vi "CRYMessages Editor.vi"() -> ()   [LabVIEW 2013]
uses:
  Typedef Control/CRYMessages Cluster.ctl
  <vilib>/Utility/miscctls.llb/LVBoundsTypeDef.ctl
  Typedef Control/CRYText Format.ctl
  CRYProject/CRYProject Editor Global.vi
  CRYWindow/SubVI/CRYMain Sub Window Global.vi
  CRYMainGlobal.vi
  CRYStepSetup/CRYStepSetup Global.vi
panel:
  in  "Digital IO Update":bool caption="对话"
  out "Message Cluster Bk":T1={"Name"="Default", "Type"=0, "Command Msg"="<Enter message or command here>", "Flags"=0, "Dialog?"=FALSE, "Numeric?"=FALSE, "Wait?"=FALSE, "Pause [ms]"=0, "pattern"=0, "Address"="", "Operation"=0, "bytes"=0, "Line selected"=0, "RS232 Func"=0, "Serial Ctrl lines"=0, "Interf #"=0, "GPIB func"=0, "GPIB cmd"=0, "GPIB rem en"=FALSE, "GPIB term"=0, "Curves generated"=[], "Units"={"unit"="", "dB ref"=0.0, "axis"=0, "data"=0, "Common dB ref."=1}, "Axis"=0, "Default Value"=0.0, "Message Tilte"="", "Port #"=0, "Print Unit"="", "Text Format"={"Size"=0, "Plain"=FALSE, "Bold"=FALSE, "Italic"=FALSE, "Underline"=FALSE, "Strikethrough"=FALSE, "Color"=0, "Font"=""}, "Help"="", "Tab Value"=enum."Setting", "pattern 2"=0, "Line selected 2"=0, "H_Bits"=[], "G_Bits"=[]} {"pattern 2" format="%.0b"; "Units"."Common dB ref." items=["dB", "dBSPL", "dBPa", "dBV", "dBm", "dBu", "dBFS"]; "Units"."dB ref" format="%.2f"; "pattern" format="%.0b"; "Flags" items=["Pass", "Fail"]}
  out "EndFlag":bool
  in  "Add Lib":bool caption="Apply"
  in  "AddStep":bool
  in  "Board Tab":enum32{"Page 1"}(tab)
  in  "Cancel":bool caption="Apply"
  in  "OK":bool caption="Apply"
  in  "Main Tab":enum32{"Setting", "Help"}(tab)
  in  "Setting":bool caption="Apply"
  in  "Line selected 2":T2={"Line"=TRUE, "Line"=TRUE, "Line"=TRUE, "Line"=TRUE, "Line"=TRUE, "Line"=TRUE, "Line"=TRUE, "Line"=TRUE} caption="Port H"
  out "Pattern 2":T3
  in  "Wait unit":string
  in  "RS-232 Func":u16(ring) caption="功能" items=["Write/Read Message", "Set Control Lines", "Read Control Lines"]
  in  "Format Text":bool
  in  "Serial Ctrl line":u16(slide) caption="Type 2"
  in  "Serial Ctrl line Read":u16(slide) caption="Type 2"
  in  "Remote Enable":bool caption="远程启用"
  in  "Command":u16(ring) caption="命令" items=["Device Clear", "Selected Device Clear", "Group Execute Trigger", "Go To Local", "Local Lockout", "Unlisten"]
  out "Interface Type":u16(ring) items=["IEEE-488", "RS-232", "Footswitch", "Buzzer"]
  in  "GPIB Function":u16(ring) caption="功能" items=["Write/Read Message", "Interface Message", "Serial Poll", "Wait for Service Request"]
  in  "Msg. term.":i32(ring) caption="项目" items=["EOI", "CR, EOI", "LF, EOI", "CR, LF, EOI", "CR", "LF", "CR, LF", "none"]
  in  "Address":i32=1 caption="地址" min=1 max=31 step=1
  in  "Bytes":i32 caption="位数"
  in  "Line selected":T2={"Line"=TRUE, "Line"=TRUE, "Line"=TRUE, "Line"=TRUE, "Line"=TRUE, "Line"=TRUE, "Line"=TRUE, "Line"=TRUE} caption="Port G"
  out "Pattern":T3
  in  "Dlg Def Val":u16(slide) caption="默认值"
  in  "Operation":i32(slide)
  in  "Dialog":bool caption="对话"
  in  "Numeric":bool caption="数字"
  in  "Wait":bool caption="等待"
  in  "Flags":u16(slide)=1
  in  "Command Msg":string="NO ELECTRICAL SIGNAL DETECTED!\nCheck wiring and connections."
  in  "Type":u16(slide)
  in  "Message Title":string caption="消息标题"
  out "DIO direction":bool=TRUE
  in  "Port":i32(ring) caption="端口"
  in  "No.":u8(ring) caption="Port"
  in  "Timeout":i32 caption="暂停" min=0 max=999999 step=1
  in  "Units Tab":enum32{"Page 1"}(tab)
  in  "Axis":u16(slide) caption="轴" scale=0.0..2.0
  out "Units":string caption="单位"
  in  "Default Value":dbl caption="默认值" format="%#.6p"
  in  "Unit Control":bool caption="Unit..."
  out "Settings":bool caption="设置"
  out "Message":bool caption="消息"
  in  "Help":string
  in  "Apply":bool
  in  "Save As...":bool caption="Apply"
  in  "Revert":bool caption="Apply"
  in  "Load...":bool caption="Apply"
  out "Interface Name":u16[](array[numeric])
  in  "Text Format":T4
  in  "Units Cluster":T5={"unit"="", "dB ref"=0.0, "axis"=0, "data"=0, "Common dB ref."=1} {"Common dB ref." items=["dB", "dBSPL", "dBPa", "dBV", "dBm", "dBu", "dBFS"]; "dB ref" format="%.2f"}
  out "DIO Array":bool[](array[boolean])
  in  "Channel":i32=-1
  in  "Calibration in":string
  in  "Hardware in":string
  in  "Load Test":bool
  out "Proper VI No":i32
  out "VIMiniumBound":T6
  out "Message Cluster":T1={"Name"="Default", "Type"=0, "Command Msg"="<Enter message or command here>", "Flags"=0, "Dialog?"=FALSE, "Numeric?"=FALSE, "Wait?"=FALSE, "Pause [ms]"=0, "pattern"=0, "Address"="", "Operation"=0, "bytes"=0, "Line selected"=0, "RS232 Func"=0, "Serial Ctrl lines"=0, "Interf #"=0, "GPIB func"=0, "GPIB cmd"=0, "GPIB rem en"=FALSE, "GPIB term"=0, "Curves generated"=[], "Units"={"unit"="", "dB ref"=0.0, "axis"=0, "data"=0, "Common dB ref."=1}, "Axis"=0, "Default Value"=0.0, "Message Tilte"="", "Port #"=0, "Print Unit"="", "Text Format"={"Size"=0, "Plain"=FALSE, "Bold"=FALSE, "Italic"=FALSE, "Underline"=FALSE, "Strikethrough"=FALSE, "Color"=0, "Font"=""}, "Help"="", "Tab Value"=enum."Setting", "pattern 2"=0, "Line selected 2"=0, "H_Bits"=[], "G_Bits"=[]} {"pattern 2" format="%.0b"; "Units"."Common dB ref." items=["dB", "dBSPL", "dBPa", "dBV", "dBm", "dBu", "dBFS"]; "Units"."dB ref" format="%.2f"; "pattern" format="%.0b"; "Flags" items=["Pass", "Fail"]}
  in  "stop":bool
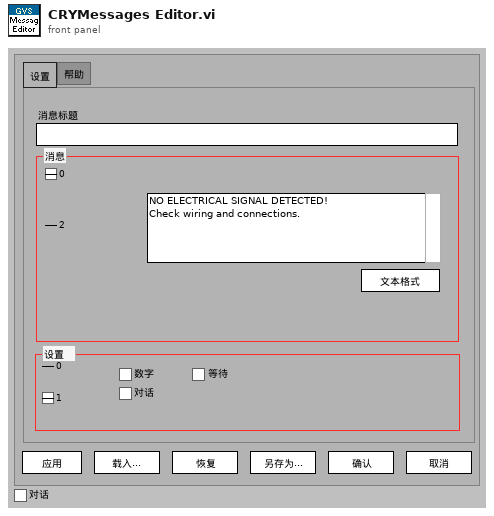
[diagram p1: front panel]
types:
  T1 = typedef "CRYMessages Cluster.ctl" = cluster{"Name":string, "Type":u16, "Command Msg":string, "Flags":u16, "Dialog?":bool, "Numeric?":bool, "Wait?":bool, "Pause [ms]":i32, "pattern":u32, "Address":string, "Operation":i32, "bytes":i32, "Line selected":u32, "RS232 Func":u16, "Serial Ctrl lines":u16, "Interf #":u8, "GPIB func":u16, "GPIB cmd":u16, "GPIB rem en":bool, "GPIB term":i32, "Curves generated":string[], "Units":cluster{"unit":string, "dB ref":dbl, "axis":u16, "data":u16, "Common dB ref.":u16}, "Axis":u16, "Default Value":dbl, "Message Tilte":string, "Port #":i32, "Print Unit":string, "Text Format":cluster{"Size":u32, "Plain":bool, "Bold":bool, "Italic":bool, "Underline":bool, "Strikethrough":bool, "Color":u32, "Font":string}, "Help":string, "Tab Value":enum32{"Setting", "Help"}, "pattern 2":u32, "Line selected 2":u32, "H_Bits":cluster{"Bits":string[], "Invert":bool, "All":bool}[], "G_Bits":cluster{"Bits":string[], "Invert":bool, "All":bool}[]}
  T2 = cluster{"Line":bool, "Line":bool, "Line":bool, "Line":bool, "Line":bool, "Line":bool, "Line":bool, "Line":bool}
  T3 = cluster{"0":bool, "1":bool, "2":bool, "3":bool, "4":bool, "5":bool, "6":bool, "7":bool}
  T4 = typedef "CRYText Format.ctl" = cluster{"Size":u32, "Plain":bool, "Bold":bool, "Italic":bool, "Underline":bool, "Strikethrough":bool, "Color":u32, "Font":string}
  T5 = cluster{"unit":string, "dB ref":dbl, "axis":u16, "data":u16, "Common dB ref.":u16}
  T6 = typedef "LVBoundsTypeDef.ctl" = cluster{"Width":u32, "Height":u32}
  T7 = typedef "CRYStep.ctl" = cluster{"No.VI":i32, "Category":string, "StepName":string, "Seq setup flattened":string, "Comment":string, "Steps config.":bool[], "Jump config":i32[], "Start":dbl, "Increment":dbl, "Name":string, "Unit":string, "Y data":u16, "Y prefix":string, "Y dB ref":dbl, "Y unit":string, "Repeat State Array":cluster{"Start":dbl, "Increment":dbl, "Count":i32, "Num":i32}[]}
  T8 = typedef "CRYHardware.ctl" = cluster{"Name":string, "Analog I/O":u16, "Digital I/O":u16, "Channels":u8, "Dig Dev ID":u8, "N ports":u8, "Interface":u32, "Dig I/O Ports":cluster{"port #":i16, "width":i16, "direction":i32}[], "Interf settings":cluster{"Type":u16, "COM Port":u8, "Baud rate":u32, "Data bits":u32, "Parity":u16, "Stop bits":u16, "Flow control":u16, "Dev ID IEEE":u8}[], "N interfs":i32, "udev SNs":i16[], "udev enable":bool, "Channel Array":T9[], "Cal sequence":string, "SelectedIn":u16, "SelectedOut":u16, "SelectedTab":u16, "State":bool, "Help":string, "Advanced":bool, "In Audio Driver":u16, "Out Audio Driver":u16}
  T9 = typedef "CRYHardware Channel Info.ctl" = cluster{"ID":i32, "Name":string, "Digital":bool, "Input":bool, "Device Name":string, "Hardware Ch ID":u8, "Vmax (V)":dbl, "Latency (samples)":dbl, "Sampling Rate (Hz)":u32, "Bit Depth":u32, "Anti-aliasing Factor (%fs)":sgl, "DAQmx Channel":tag, "term config":i32, "Coupling":i32, "IEPE en":bool, "ASIOChannel Name":string, "Audio Driver":u16, "ASIOChannel Index":u8}
  T10 = cluster{"port #":i16, "width":i16, "direction":i32}[]
  T11 = cluster{"Type":u16, "COM Port":u8, "Baud rate":u32, "Data bits":u32, "Parity":u16, "Stop bits":u16, "Flow control":u16, "Dev ID IEEE":u8}[]
  T12 = enum16{"OK", "Yes", "YesNo", "YesNoCancel", "ReplaceAppend"}
  T13 = enum8{"Enabled", "Disabled", "Disabled and Grayed Out"}
  T14 = cluster{"Bits":string[], "Invert":bool, "All":bool}[]
  T15 = cluster{"Load Test":bool, "Format Text":bool, "Unit Control":bool, "Apply":bool, "Add Lib":bool, "OK":bool, "Cancel":bool, "Setting":bool}
  T16 = cluster{"Size":u32, "Plain":bool, "Bold":bool, "Italic":bool, "Underline":bool, "Strikethrough":bool, "Color":u32, "Font":string}
  T17 = cluster{"Boolean array[0]":bool, "Boolean array[1]":bool, "Boolean array[2]":bool, "Boolean array[3]":bool, "Boolean array[4]":bool, "Boolean array[5]":bool, "Boolean array[6]":bool, "Boolean array[7]":bool}
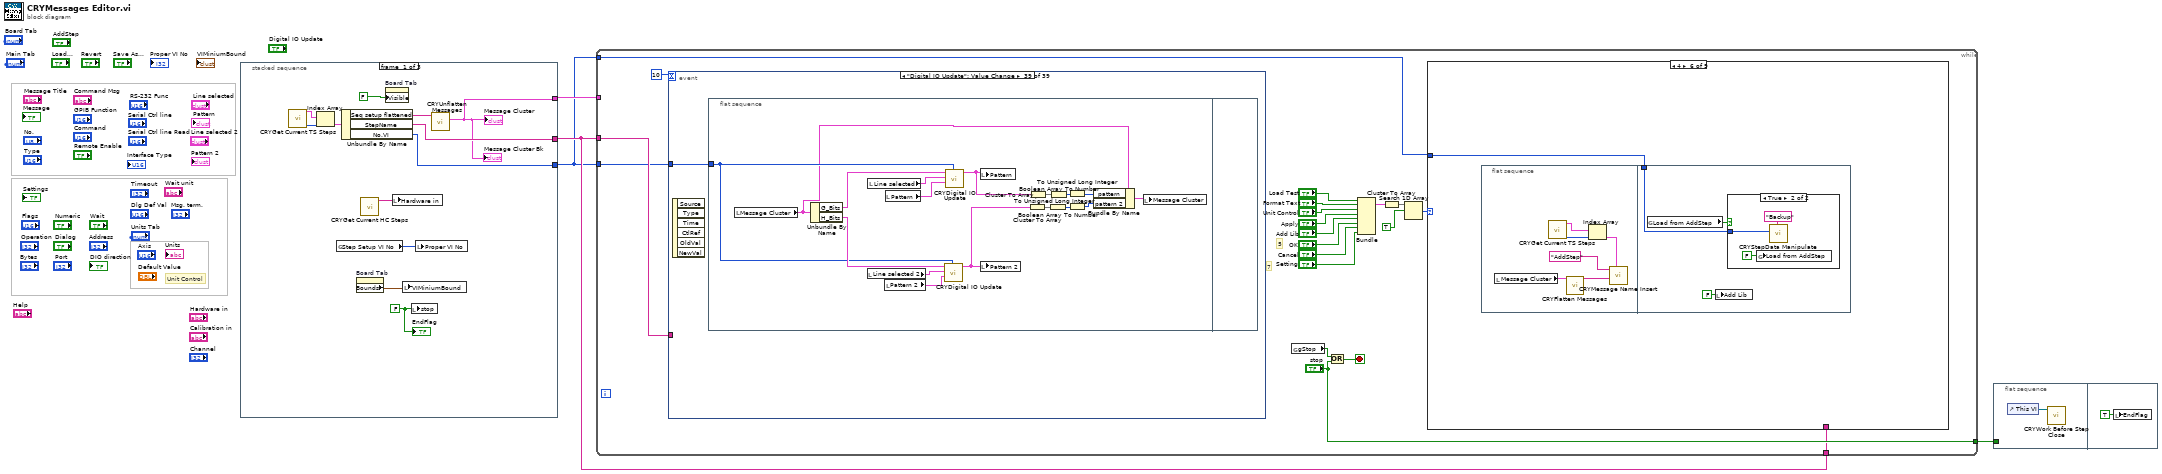
[diagram p0: block diagram]
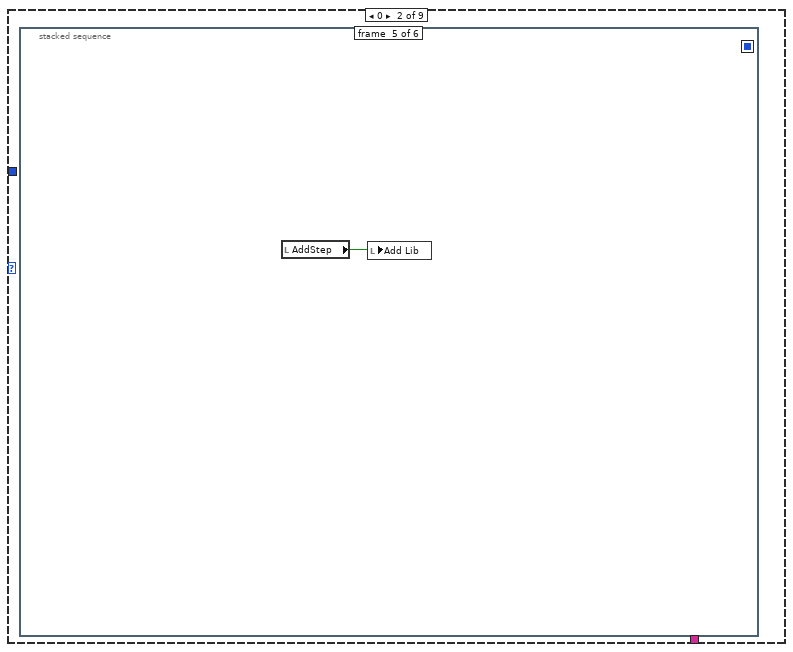
[diagram p3: hidden frame]
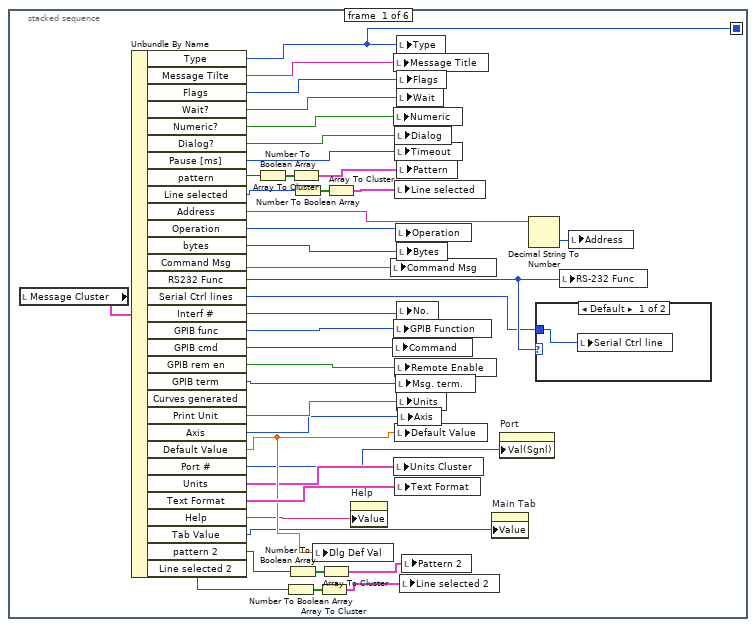
[diagram p4: hidden frame]
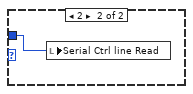
[diagram p5: hidden frame]
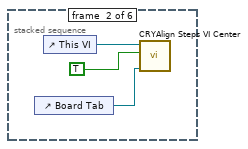
[diagram p6: hidden frame]
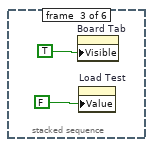
[diagram p7: hidden frame]
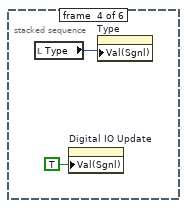
[diagram p8: hidden frame]
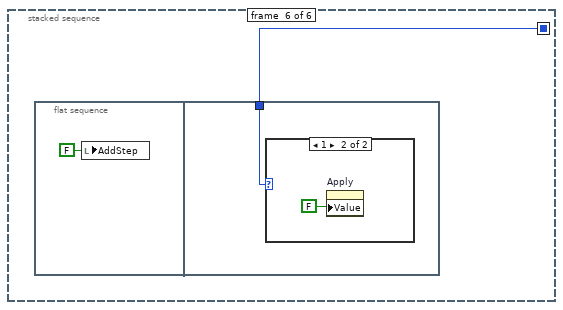
[diagram p9: hidden frame]
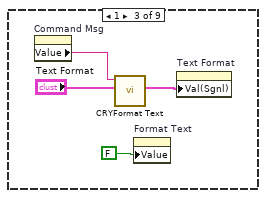
[diagram p11: hidden frame]
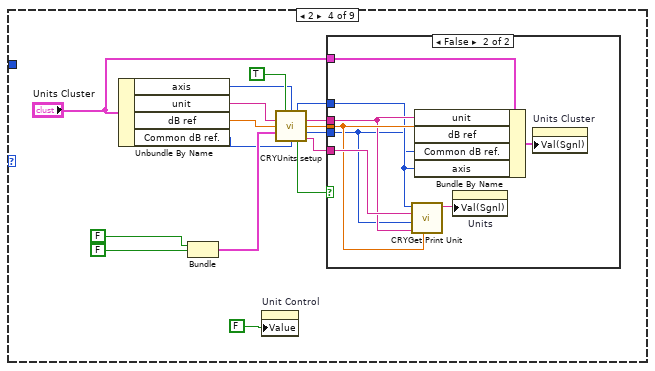
[diagram p12: hidden frame]
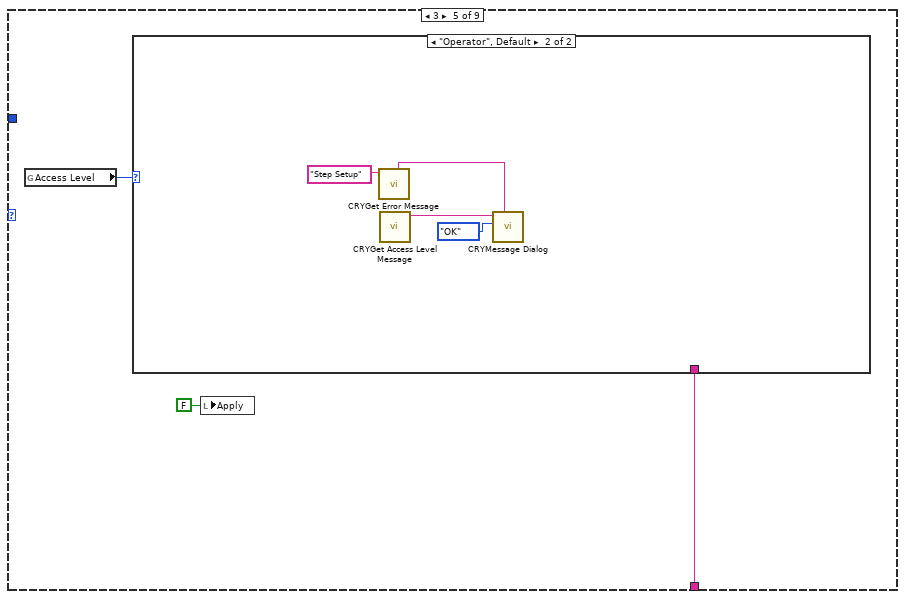
[diagram p14: hidden frame]
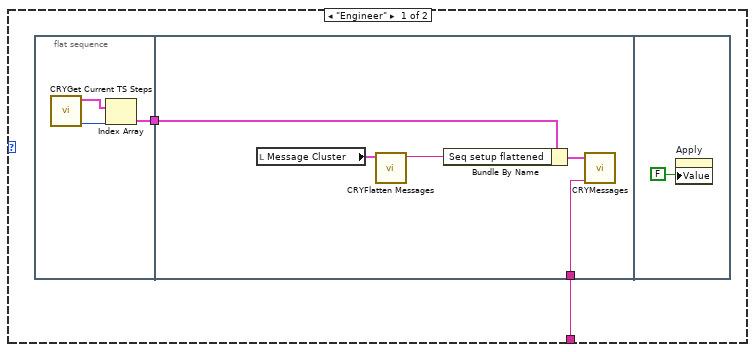
[diagram p15: hidden frame]
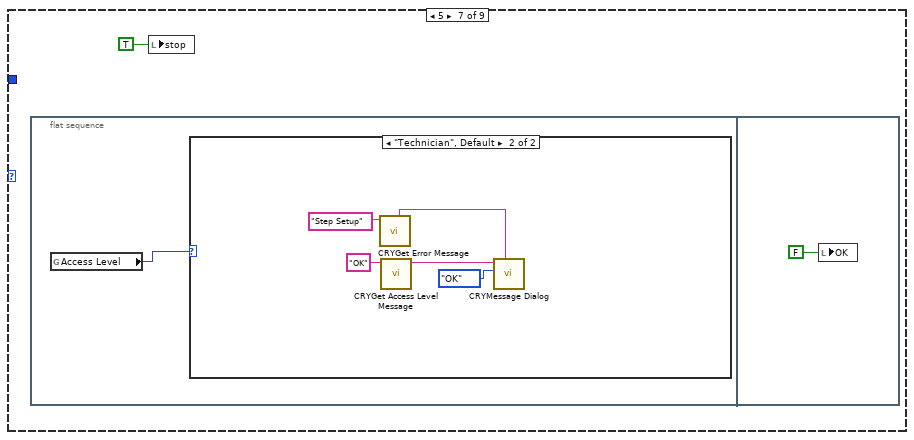
[diagram p17: hidden frame]
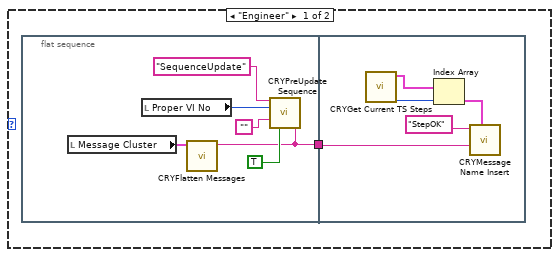
[diagram p18: hidden frame]
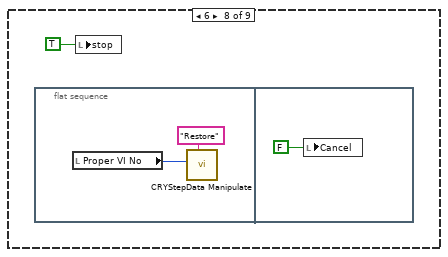
[diagram p19: hidden frame]
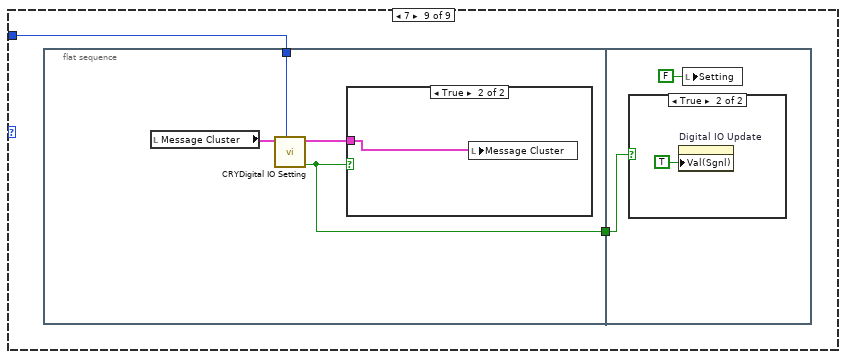
[diagram p20: hidden frame]
diagram:
  # "Unit Control"
  n1 = stacked-sequence {
    tunnel: [w7 _ _] -> w4
    tunnel: [w8 _ _] -> w2
    tunnel: [w5 _ _] -> w1
    frame #0 {
      w6 = FALSE ("stop")
      n2 = call "CRYGet Current TS Steps.vi"() -> ("SelectStepNumber in Tree"=w12:i32, "Steps"=w13:T7[])  [unwired: 1 in, 9 out]
      n3 = Index Array(array=w13, index=w12) -> (element=w16:T7)
      n4 = global read "CRYProject Editor Global.vi" "Step Setup VI No"() -> (w14:i32)
      n5 = Unbundle By Name(w16) -> ("Seq setup flattened"=w15:string, "StepName"=w8:string, "No.VI"=w5:i32)
      n6 = property on="Board Tab" class="TabCtl (strict)"() -> ("Bounds"=w10:T6)  [unwired: 2 in, 2 out]
      n7 = call "CRYGet Current HC Steps.vi"() -> ("Hardware setup flattened Out"=w9:string)  [unwired: 10 in, 1 out]
      n8 = property on="Board Tab" class="TabCtl (strict)"("Visible"=FALSE) -> ()  [unwired: 2 in, 2 out]
      n9 = local write "Hardware in"(w9) -> ()
      n10 = local write "VIMiniumBound"(w10) -> ()
      n11 = local write "stop"(w6) -> ()
      n12 = local write "Proper VI No"(w14) -> ()
      n13 = call "CRYUnflatten Messages.vi"("Unflatten Messages"=w15) -> ("Messages"=w7:T1)  [unwired: 10 out]
      "Message Cluster" <- w7
      "Message Cluster Bk" <- w7
      "EndFlag" <- w6
    }
    frame #1 {
      w19 = FALSE ("Visible")
      n14 = local read "Hardware in"() -> (w26:string)
      n15 = call "CRYUnflatten SoundCard.vi"("Flatten SoundCard"=w26) -> ("SoundCard"=w29:T8)  [unwired: 10 out]
      n16 = local write "Wait unit"("ms" ("Wait unit")) -> ()
      n17 = Unbundle By Name(w29) -> ("N ports"=w28:u8, "Dig I/O Ports"=w23:T10, "N interfs"=w20:i32, "Interf settings"=w25:T11)
      n18 = property on="Unit Control" class="Bool (strict)"("Value"=w19) -> ()  [unwired: 2 in, 2 out]
      n19 = local write "Default Value"(0.0 ("Default Value")) -> ()
      n20 = for {
        N: w20 -> [_]
        tunnel: [w32] -> w27 mode=indexing
        tunnel: w25 -> [w31] mode=indexing
        tunnel: [w30] -> w24 mode=indexing
        i -> [w34]
        n21 = Increment(x=w34) -> (x+1=w33:i32)
        n22 = Unbundle By Name(w31) -> ("Type"=w30:u16)
        n23 = Number To Decimal String(number=w33) -> (decimal integer string=w32:string)  [unwired: 1 out]
      }
      "Interface Name" <- w24
      n24 = for {
        N: w28 -> [_]
        tunnel: [w38] -> w21 mode=indexing
        tunnel: w23 -> [w36] mode=indexing
        tunnel: [w35] -> w22 mode=indexing
        i -> [w40]
        n25 = Increment(x=w40) -> (x+1=w39:i32)
        n26 = Unbundle By Name(w36) -> ("direction"=w37:i32)
        n27 = Number To Decimal String(number=w39) -> (decimal integer string=w38:string)  [unwired: 1 out]
        n28 = Not Equal To 0?(x=w37) -> (x != 0?=w35:bool)
      }
      "DIO Array" <- w22
      n29 = property on="Format Text" class="Bool (strict)"("Value"=w19) -> ()  [unwired: 2 in, 2 out]
      n30 = property on="Apply" class="Bool (strict)"("Value"=w19) -> ()  [unwired: 2 in, 2 out]
      n31 = property on="No." class="Ring (strict)"("Strings []"=w27) -> ()  [unwired: 2 in, 2 out]
      n32 = property on="Port" class="Ring (strict)"("Strings []"=w21) -> ()  [unwired: 2 in, 2 out]
    }
    frame #2 {
      n33 = property on="Load Test" class="Bool (strict)"("Value"=TRUE ("Load Test")) -> ()  [unwired: 2 in, 2 out]
    }
  }
  n34 = while {
    tunnel: w4 -> [_]
    tunnel: ["stop"] -> w3
    tunnel: w2 -> [w49]
    tunnel: w2 -> [w48]
    tunnel: w1 -> [w43]
    tunnel: w1 -> [w42]
    stop <- w52 stop-if-true
    # "7"
    # "5"
    n35 = event shown="[38] \"Digital IO Update\": Value Change" {
      selector: _ -> [_ _ _ _ _ _ _ _ _ _ _ _ _ _ _ _ _ _ _ _ _ _ _ _ _ _ _ _ _ _ _ _ _ _ _ _ _ _ _]
      dyn-events: _ -> [_ _ _ _ _ _ _ _ _ _ _ _ _ _ _ _ _ _ _ _ _ _ _ _ _ _ _ _ _ _ _ _ _ _ _ _ _ _ _]
      timeout: 10 -> [_ _ _ _ _ _ _ _ _ _ _ _ _ _ _ _ _ _ _ _ _ _ _ _ _ _ _ _ _ _ _ _ _ _ _ _ _ _ _]
      tunnel: w49 -> [_ _ _ _ _ _ w263 w309 w321 _ w346 _ w382 w402 _ _ _ _ _ _ _ _ _ _ _ _ _ _ w497 _ _ _ _ _ _ _ _ _ _]
      tunnel: w43 -> [_ _ _ _ _ _ _ _ _ _ _ _ _ _ _ _ _ _ _ _ _ _ _ _ _ _ _ _ _ _ _ _ _ _ _ _ _ _ w560]
      event Timeout {
        n36 = event-data() -> ()  [unwired: 3 out]
      }
      event Pane Size {
        n37 = event-data() -> ()  [unwired: 7 out]
        n38 = control-ref of="Board Tab"() -> (w209:refnum<vi>)
        n39 = control-ref of="This VI"() -> (w211:refnum<vi>)
        n40 = call "CRYAlign Steps VI Center.vi"("Tab2"=w209, "Input/Output"=TRUE, "VIRef"=w211) -> ()  [unwired: 1 in, 8 out]
      }
      event "Load...": Value Change {
        n41 = event-data() -> ("CtlRef"=w212:refnum<vi>)  [unwired: 6 out]
        n42 = property on="Load Test" class="Bool (strict)"() -> ("Value"=w214:bool)  [unwired: 2 in, 2 out]
        n43 = property class="Bool (strict)"(reference=w212, "Value"=FALSE) -> ()  [unwired: 1 in, 2 out]
        n44 = case shown="False" w214 {
          frame False {
            n45 = global read "CRYMainGlobal.vi" "Steps path"() -> (w219:path)
            n46 = local read "Proper VI No"() -> (w215:i32)
            n47 = Build Path(base path=w219, name or relative path="CRYMessages") -> (appended path=w220:path)
            n48 = call "CRYStep Read.vi"("Category Name"="Messages" ("Step File Name"), "Proper VI No"=w215, "Step File Path"=w220) -> ("status"=w221:bool, "selected path"=w216:path, "Flatten Step"=w222:string)  [unwired: 1 in, 3 out]
            n49 = case shown="True" w221 {
              tunnel: w222 -> [_ w224]
              tunnel: w216 -> [_ w225]
              tunnel: w215 -> [_ w223]
              frame False {
              }
              frame True {
                n50 = call "CRYUnflatten Messages.vi"("Unflatten Messages"=w224) -> ("Error?"=w226:bool, "Messages"=w227:T1)  [unwired: 9 out]
                n51 = case shown="False" w226 {
                  tunnel: w227 -> [w231 _]
                  tunnel: w225 -> [w230 _]
                  tunnel: w224 -> [w229 _]
                  tunnel: w223 -> [w228 _]
                  frame False {
                    n52 = flat-sequence {
                      tunnel: w231 -> [w243]
                      tunnel: w230 -> [w239]
                      tunnel: w229 -> [w237]
                      tunnel: w228 -> [w238]
                      frame #0 {
                        n53 = local write "Message Cluster"(w243) -> ()
                        n54 = Strip Path(path=w239) -> (name=w233:string)  [unwired: 1 out]
                        n55 = Reverse String(1:w233) -> (0:w235:string)
                        n56 = Match Pattern(string=w235, regular expression="[.]") -> (after substring=w236:string)  [unwired: 4 out]
                        n57 = Reverse String(1:w236) -> (0:w232:string)
                        n58 = call "CRYPreUpdate Sequence.vi"("EventName"="Load", "StepName Arg3"=w232, "Proper VI No"=w238, "Project View Step Name Identifier Arg1"="", "Step flattened Arg2"=w237, "AllChangeFlg"=TRUE ("Name/Identifier")) -> ()  [unwired: 10 in]
                      }
                      frame #1 {
                        n59 = local write "Load Test"(TRUE ("Load Test")) -> ()
                      }
                    }
                  }
                  frame True {
                  }
                }
              }
            }
          }
          frame True {
          }
        }
      }
      event "Save As...": Value Change {
        w247 = "Messages" ("Step File Name")
        n60 = event-data() -> ("CtlRef"=w245:refnum<vi>)  [unwired: 6 out]
        n61 = property class="Bool (strict)"(reference=w245, "Value"=FALSE) -> ()  [unwired: 1 in, 2 out]
        n62 = local read "Message Cluster"() -> (w255:T1)
        n63 = global read "CRYMainGlobal.vi" "Steps path"() -> (w248:path)
        n64 = call "CRYFlatten Messages.vi"("Messages"=w255) -> ("Flatten Messages String"=w249:string)  [unwired: 10 out]
        n65 = local read "Proper VI No"() -> (w250:i32)
        n66 = Build Path(base path=w248, name or relative path="CRYMessages") -> (appended path=w252:path)
        n67 = call "CRYStep Write.vi"("StepIdentifier"="", "Default"=FALSE, "Proper VI No"=w250, "Category Name"=w247, "Step File Path"=w252, "Step flattened"=w249, "Step File Name"=w247) -> ()  [unwired: 1 in, 4 out]
      }
      event "Revert": Value Change {
        n68 = event-data() -> ("CtlRef"=w257:refnum<vi>)  [unwired: 6 out]
        n69 = flat-sequence {
          frame #0 {
            n70 = local read "Message Cluster Bk"() -> (w258:T1)
            n71 = local write "Message Cluster"(w258) -> ()
          }
          frame #1 {
            n72 = local write "Load Test"(TRUE ("Load Test")) -> ()
          }
        }
        n73 = property class="Bool (strict)"(reference=w257, "Value"=FALSE) -> ()  [unwired: 1 in, 2 out]
      }
      event Panel Close {
        n74 = event-data() -> ()  [unwired: 5 out]
        n75 = control-ref of="This VI"() -> (w261:refnum<vi>)
        n76 = local write "Cancel"(TRUE ("Cancel")) -> ()
        n77 = call "CRYWork Before Step Close.vi"("StepVI Ref"=w261) -> ()  [unwired: 11 in]
      }
      event "Type": Value Change {
        n78 = event-data() -> ("NewVal"=w264:u16)  [unwired: 6 out]
        n79 = local read "Interface Type"() -> (w271:u16)
        n80 = local read "RS-232 Func"() -> (w270:u16)
        n81 = local read "Operation"() -> (w269:i32)
        n82 = local read "Numeric"() -> (w267:bool)
        n83 = local read "Dialog"() -> (w268:bool)
        n84 = local read "GPIB Function"() -> (w272:u16)
        n85 = case shown="1" w264 {
          tunnel: [FALSE TRUE FALSE] -> w262
          frame 0, Default {
            w275 = FALSE
            w291 = TRUE ("Visible")
            n86 = local read "Numeric"() -> (w289:bool)
            n87 = local read "Dialog"() -> (w290:bool)
            n88 = property on="DIO direction" class="Bool (strict)"("Visible"=w275) -> ()  [unwired: 2 in, 2 out]
            n89 = property on="Pattern" class="Clust (strict)"("Visible"=w275) -> ()  [unwired: 2 in, 2 out]
            n90 = property on="Command Msg" class="Str"("Visible"=w291) -> ()  [unwired: 2 in, 2 out]
            n91 = property on="Flags" class="Slide (strict)"("Visible"=w291) -> ()  [unwired: 2 in, 2 out]
            n92 = Equal?(x=w290, y=FALSE) -> (x = y?=w284:bool)
            n93 = Equal?(x=w289, y=FALSE) -> (x = y?=w285:bool)
            n94 = property on="Line selected" class="Clust (strict)"("Visible"=w275) -> ()  [unwired: 2 in, 2 out]
            n95 = property on="Wait" class="Bool (strict)"("Visible"=w291) -> ()  [unwired: 2 in, 2 out]
            n96 = Not(x=w285) -> (.not. x?=w283:bool)
            n97 = property on="Port" class="Ring (strict)"("Visible"=w275) -> ()  [unwired: 2 in, 2 out]
            n98 = Not(x=w284) -> (.not. x?=w286:bool)
            n99 = property on="Format Text" class="Bool (strict)"("Visible"=w291) -> ()  [unwired: 2 in, 2 out]
            n100 = And(x=w284, y=w285) -> (x .and. y?=w279:bool)
            n101 = And(x=w286, y=w285) -> (x .and. y?=w278:bool)
            n102 = And(x=w284, y=w283) -> (x .and. y?=w277:bool)
            n103 = property on="Command" class="Ring (strict)"("Visible"=w275) -> ()  [unwired: 2 in, 2 out]
            n104 = property on="No." class="Ring (strict)"("Visible"=w275) -> ()  [unwired: 2 in, 2 out]
            n105 = property on="Numeric" class="Bool (strict)"("Visible"=w291) -> ()  [unwired: 2 in, 2 out]
            n106 = Bundle(w279, w278, w277) -> (w281:cluster{bool, bool, bool})  [unwired: 1 out]
            n107 = property on="Remote Enable" class="Bool (strict)"("Visible"=w275) -> ()  [unwired: 2 in, 2 out]
            n108 = property on="Interface Type" class="Ring (strict)"("Visible"=w275) -> ()  [unwired: 2 in, 2 out]
            n109 = Cluster To Array(cluster=w281) -> (array=w280:bool[])
            n110 = property on="Dialog" class="Bool (strict)"("Visible"=w291) -> ()  [unwired: 2 in, 2 out]
            n111 = Search 1D Array(1D array=w280, element=TRUE) -> (index of element=w276:i32)  [unwired: 1 out]
            n112 = property on="RS-232 Func" class="Ring (strict)"("Visible"=w275) -> ()  [unwired: 2 in, 2 out]
            n113 = property on="GPIB Function" class="Ring (strict)"("Visible"=w275) -> ()  [unwired: 2 in, 2 out]
            n114 = case shown="0, 2, Default" w276 {
              frame 0, 2, Default {
                n115 = local read "Numeric"() -> (w293:bool)
                n116 = property on="Numeric" class="Bool (strict)"("Disabled"=u8 0, "Val(Sgnl)"=w293) -> ()  [unwired: 2 in, 2 out]
              }
              frame 1 {
                n117 = local read "Dialog"() -> (w295:bool)
                n118 = property on="Dialog" class="Bool (strict)"("Disabled"=u8 0, "Val(Sgnl)"=w295) -> ()  [unwired: 2 in, 2 out]
              }
            }
            n119 = property on="Address" class="DigNum (strict)"("Visible"=w275) -> ()  [unwired: 2 in, 2 out]
            n120 = property on="Serial Ctrl line" class="Slide (strict)"("Visible"=w275) -> ()  [unwired: 2 in, 2 out]
            n121 = property on="Operation" class="Slide (strict)"("Visible"=w275) -> ()  [unwired: 2 in, 2 out]
            n122 = property on="Line selected 2" class="Clust (strict)"("Visible"=w275) -> ()  [unwired: 2 in, 2 out]
            n123 = property on="Bytes" class="DigNum (strict)"("Visible"=w275) -> ()  [unwired: 2 in, 2 out]
            n124 = property on="Serial Ctrl line Read" class="Slide (strict)"("Visible"=w275) -> ()  [unwired: 2 in, 2 out]
            n125 = property on="Msg. term." class="Ring (strict)"("Visible"=w275) -> ()  [unwired: 2 in, 2 out]
            n126 = property on="Pattern 2" class="Clust (strict)"("Visible"=w275) -> ()  [unwired: 2 in, 2 out]
          }
          frame 1 {
            w298 = FALSE ("Visible")
            w297 = TRUE ("Visible")
            n127 = property on="Flags" class="Slide (strict)"("Visible"=w297) -> ()  [unwired: 2 in, 2 out]
            n128 = property on="Pattern" class="Clust (strict)"("Visible"=w297) -> ()  [unwired: 2 in, 2 out]
            n129 = property on="Command Msg" class="Str"("Visible"=w298) -> ()  [unwired: 2 in, 2 out]
            n130 = property on="Dlg Def Val" class="Slide (strict)"("Visible"=w298) -> ()  [unwired: 2 in, 2 out]
            n131 = property on="RS-232 Func" class="Ring (strict)"("Visible"=w298) -> ()  [unwired: 2 in, 2 out]
            n132 = property on="GPIB Function" class="Ring (strict)"("Visible"=w298) -> ()  [unwired: 2 in, 2 out]
            n133 = property on="DIO direction" class="Bool (strict)"("Visible"=w298) -> ()  [unwired: 2 in, 2 out]
            n134 = property on="Line selected" class="Clust (strict)"("Visible"=w297) -> ()  [unwired: 2 in, 2 out]
            n135 = property on="Units Tab" class="TabCtl (strict)"("Visible"=w298) -> ()  [unwired: 2 in, 2 out]
            n136 = property on="Serial Ctrl line" class="Slide (strict)"("Visible"=w298) -> ()  [unwired: 2 in, 2 out]
            n137 = property on="Operation" class="Slide (strict)"("Visible"=w298) -> ()  [unwired: 2 in, 2 out]
            n138 = property on="Port" class="Ring (strict)"("Visible"=w298) -> ()  [unwired: 2 in, 2 out]
            n139 = property on="Format Text" class="Bool (strict)"("Visible"=w298) -> ()  [unwired: 2 in, 2 out]
            n140 = property on="Address" class="DigNum (strict)"("Visible"=w298) -> ()  [unwired: 2 in, 2 out]
            n141 = property on="Command" class="Ring (strict)"("Visible"=w298) -> ()  [unwired: 2 in, 2 out]
            n142 = property on="Line selected 2" class="Clust (strict)"("Visible"=w297) -> ()  [unwired: 2 in, 2 out]
            n143 = property on="Bytes" class="DigNum (strict)"("Visible"=w298) -> ()  [unwired: 2 in, 2 out]
            n144 = property on="Numeric" class="Bool (strict)"("Visible"=w298) -> ()  [unwired: 2 in, 2 out]
            n145 = property on="Serial Ctrl line Read" class="Slide (strict)"("Visible"=w298) -> ()  [unwired: 2 in, 2 out]
            n146 = property on="Msg. term." class="Ring (strict)"("Visible"=w298) -> ()  [unwired: 2 in, 2 out]
            n147 = property on="Remote Enable" class="Bool (strict)"("Visible"=w298) -> ()  [unwired: 2 in, 2 out]
            n148 = property on="Dialog" class="Bool (strict)"("Visible"=w298) -> ()  [unwired: 2 in, 2 out]
            n149 = property on="No." class="Ring (strict)"("Visible"=w298) -> ()  [unwired: 2 in, 2 out]
            n150 = property on="Pattern 2" class="Clust (strict)"("Visible"=w297) -> ()  [unwired: 2 in, 2 out]
            n151 = property on="Interface Type" class="Ring (strict)"("Visible"=w298) -> ()  [unwired: 2 in, 2 out]
            n152 = disable-structure shown="Disabled" {
              frame Disabled {
                n153 = local read "Wait"() -> (w301:bool)
                n154 = property on="Wait" class="Bool (strict)"("Val(Sgnl)"=w301, "DisabledEnum"=T13."Enabled" ("Disabled")) -> ()  [unwired: 2 in, 2 out]
              }
              frame Enabled {
              }
            }
            n155 = local read "Port"() -> (w299:i32)
            n156 = property on="Wait" class="Bool (strict)"("Visible"=w298) -> ()  [unwired: 2 in, 2 out]
            n157 = property on="Port" class="Ring (strict)"("Val(Sgnl)"=w299) -> ()  [unwired: 2 in, 2 out]
            n158 = property on="Timeout" class="DigNum (strict)"("Visible"=w298) -> ()  [unwired: 2 in, 2 out]
            n159 = property on="Wait unit" class="Str"("Visible"=w298) -> ()  [unwired: 2 in, 2 out]
          }
          frame 2 {
            w303 = FALSE
            w304 = TRUE ("Visible")
            n160 = property on="Flags" class="Slide (strict)"("Visible"=w304) -> ()  [unwired: 2 in, 2 out]
            n161 = property on="Numeric" class="Bool (strict)"("Visible"=w303) -> ()  [unwired: 2 in, 2 out]
            n162 = property on="Pattern" class="Clust (strict)"("Visible"=w303) -> ()  [unwired: 2 in, 2 out]
            n163 = property on="Line selected 2" class="Clust (strict)"("Visible"=w303) -> ()  [unwired: 2 in, 2 out]
            n164 = property on="Line selected" class="Clust (strict)"("Visible"=w303) -> ()  [unwired: 2 in, 2 out]
            n165 = property on="No." class="Ring (strict)"("Visible"=w304) -> ()  [unwired: 2 in, 2 out]
            n166 = property on="Dialog" class="Bool (strict)"("Visible"=w303) -> ()  [unwired: 2 in, 2 out]
            n167 = property on="Pattern 2" class="Clust (strict)"("Visible"=w303) -> ()  [unwired: 2 in, 2 out]
            n168 = property on="Dlg Def Val" class="Slide (strict)"("Visible"=w303) -> ()  [unwired: 2 in, 2 out]
            n169 = property on="Interface Type" class="Ring (strict)"("Visible"=w304) -> ()  [unwired: 2 in, 2 out]
            n170 = property on="DIO direction" class="Bool (strict)"("Visible"=w303) -> ()  [unwired: 2 in, 2 out]
            n171 = property on="Units Tab" class="TabCtl (strict)"("Visible"=w303) -> ()  [unwired: 2 in, 2 out]
            n172 = property on="Timeout" class="DigNum (strict)"("Visible"=w304) -> ()  [unwired: 2 in, 2 out]
            n173 = property on="Port" class="Ring (strict)"("Visible"=w303) -> ()  [unwired: 2 in, 2 out]
            n174 = local read "No."() -> (w308:u8)
            n175 = property on="Wait unit" class="Str"("Visible"=w304) -> (error out=w305:errorcluster)  [unwired: 2 in, 1 out]
            n176 = property on="No." class="Ring (strict)"("Val(Sgnl)"=w308) -> ()  [unwired: 2 in, 2 out]
            n177 = local read "Wait"() -> (w307:bool)
            n178 = property on="Wait" class="Bool (strict)"(error in=w305, "Val(Sgnl)"=w307, "DisabledEnum"=T13."Enabled" ("Disabled"), "Visible"=w304) -> ()  [unwired: 1 in, 2 out]
          }
        }
        n179 = call "CRYMsgs Curves Gen Construct.vi"("Interface type"=w271, "GPIB func"=w272, "Step name"=w263, "Type"=w264, "RS232 func"=w270, "Operation"=w269, "Numeric?"=w267, "Dialog?"=w268) -> ("Curves generated"=w266:string[])  [unwired: 3 in]
        n180 = local read "Message Cluster"() -> (w273:T1)
        n181 = Bundle By Name(cluster=w273, "Type"=w264, "Curves generated"=w266) -> (w265:T1)
        n182 = local write "Message Cluster"(w265) -> ()
        n183 = property on="Setting" class="Bool (strict)"("Visible"=w262) -> ()  [unwired: 2 in, 2 out]
      }
      event "GPIB Function": Value Change {
        n184 = event-data() -> ("NewVal"=w314:u16)  [unwired: 6 out]
        n185 = local read "Interface Type"() -> (w319:u16)
        n186 = local read "RS-232 Func"() -> (w318:u16)
        n187 = local read "Operation"() -> (w317:i32)
        n188 = local read "Numeric"() -> (w315:bool)
        n189 = local read "Dialog"() -> (w316:bool)
        n190 = local read "Type"() -> (w313:u16)
        n191 = call "CRYMsgs Curves Gen Construct.vi"("Interface type"=w319, "GPIB func"=w314, "Step name"=w309, "Type"=w313, "RS232 func"=w318, "Operation"=w317, "Numeric?"=w315, "Dialog?"=w316) -> ("Curves generated"=w312:string[])  [unwired: 3 in]
        n192 = local read "Operation"() -> (w311:i32)
        n193 = local read "Message Cluster"() -> (w320:T1)
        n194 = Bundle By Name(cluster=w320, "GPIB func"=w314, "Curves generated"=w312) -> (w310:T1)
        n195 = property on="Operation" class="Slide (strict)"("Val(Sgnl)"=w311) -> ()  [unwired: 2 in, 2 out]
        n196 = local write "Message Cluster"(w310) -> ()
      }
      event "RS-232 Func": Value Change {
        n197 = event-data() -> ("NewVal"=w324:u16)  [unwired: 6 out]
        n198 = case shown="2" w324 {
          frame 0, Default {
            n199 = stacked-sequence {
              frame #0 {
                w333 = FALSE
                w332 = TRUE
                n200 = property on="Serial Ctrl line" class="Slide (strict)"("Visible"=w333) -> ()  [unwired: 2 in, 2 out]
                n201 = property on="Serial Ctrl line Read" class="Slide (strict)"("Visible"=w333) -> ()  [unwired: 2 in, 2 out]
                n202 = property on="Command Msg" class="Str"("Visible"=w332) -> ()  [unwired: 2 in, 2 out]
                n203 = property on="Operation" class="Slide (strict)"("Visible"=w332) -> ()  [unwired: 2 in, 2 out]
                n204 = property on="Timeout" class="DigNum (strict)"("Visible"=w332, "Caption.Visible"=w332) -> ()  [unwired: 2 in, 2 out]
              }
              frame #1 {
                n205 = local read "Operation"() -> (w334:i32)
                n206 = property on="Operation" class="Slide (strict)"("Val(Sgnl)"=w334) -> ()  [unwired: 2 in, 2 out]
              }
            }
          }
          frame 1 {
            n207 = stacked-sequence {
              frame #0 {
                w336 = TRUE
                w337 = FALSE
                n208 = property on="Serial Ctrl line" class="Slide (strict)"("Visible"=w336) -> ()  [unwired: 2 in, 2 out]
                n209 = property on="Command Msg" class="Str"("Visible"=w337) -> ()  [unwired: 2 in, 2 out]
                n210 = property on="Operation" class="Slide (strict)"("Visible"=w337) -> ()  [unwired: 2 in, 2 out]
                n211 = property on="Serial Ctrl line Read" class="Slide (strict)"("Visible"=w337) -> ()  [unwired: 2 in, 2 out]
                n212 = property on="Wait" class="Bool (strict)"("Visible"=w336, "DisabledEnum"=T13."Enabled" ("Disabled")) -> ()  [unwired: 2 in, 2 out]
              }
              frame #1 {
                n213 = local read "Wait"() -> (w338:bool)
                n214 = property on="Wait" class="Bool (strict)"("Val(Sgnl)"=w338) -> ()  [unwired: 2 in, 2 out]
              }
            }
          }
          frame 2 {
            n215 = stacked-sequence {
              frame #0 {
                w340 = TRUE
                w341 = FALSE
                n216 = property on="Serial Ctrl line Read" class="Slide (strict)"("Visible"=w340) -> ()  [unwired: 2 in, 2 out]
                n217 = property on="Command Msg" class="Str"("Visible"=w341) -> ()  [unwired: 2 in, 2 out]
                n218 = property on="Operation" class="Slide (strict)"("Visible"=w341) -> ()  [unwired: 2 in, 2 out]
                n219 = property on="Serial Ctrl line" class="Slide (strict)"("Visible"=w341) -> ()  [unwired: 2 in, 2 out]
                n220 = property on="Wait" class="Bool (strict)"("Visible"=w340, "DisabledEnum"=T13."Enabled" ("Disabled")) -> ()  [unwired: 2 in, 2 out]
              }
              frame #1 {
                n221 = local read "Wait"() -> (w342:bool)
                n222 = property on="Wait" class="Bool (strict)"("Val(Sgnl)"=w342) -> ()  [unwired: 2 in, 2 out]
              }
            }
          }
        }
        n223 = local read "Interface Type"() -> (w328:u16)
        n224 = local read "GPIB Function"() -> (w329:u16)
        n225 = local read "Operation"() -> (w327:i32)
        n226 = local read "Numeric"() -> (w325:bool)
        n227 = local read "Dialog"() -> (w326:bool)
        n228 = local read "Type"() -> (w330:u16)
        n229 = call "CRYMsgs Curves Gen Construct.vi"("Interface type"=w328, "GPIB func"=w329, "Step name"=w321, "Type"=w330, "RS232 func"=w324, "Operation"=w327, "Numeric?"=w325, "Dialog?"=w326) -> ("Curves generated"=w323:string[])  [unwired: 3 in]
        n230 = local read "Message Cluster"() -> (w331:T1)
        n231 = Bundle By Name(cluster=w331, "RS232 Func"=w324, "Curves generated"=w323) -> (w322:T1)
        n232 = local write "Message Cluster"(w322) -> ()
      }
      event "Flags": Value Change {
        n233 = event-data() -> ("NewVal"=w344:u16)  [unwired: 6 out]
        n234 = local read "Message Cluster"() -> (w345:T1)
        n235 = Bundle By Name(cluster=w345, "Flags"=w344) -> (w343:T1)
        n236 = local write "Message Cluster"(w343) -> ()
      }
      event "Numeric": Value Change {
        n237 = event-data() -> ("NewVal"=w349:bool)  [unwired: 6 out]
        n238 = case shown="True" w349 {
          selector: w349 -> [w358 w367]
          frame False {
            w360 = u8 0 ("Disabled")
            n239 = property on="Units Tab" class="TabCtl (strict)"("Visible"=w358) -> ()  [unwired: 2 in, 2 out]
            n240 = property on="Dialog" class="Bool (strict)"("Disabled"=w360, "Value"=FALSE ("Dialog")) -> ()  [unwired: 2 in, 2 out]
            n241 = property on="Dlg Def Val" class="Slide (strict)"("Visible"=w358) -> ()  [unwired: 2 in, 2 out]
            n242 = property on="Wait" class="Bool (strict)"("Disabled"=w360) -> ("Value"=w357:bool)  [unwired: 2 in, 2 out]
            n243 = property on="Timeout" class="DigNum (strict)"("Visible"=w357) -> ()  [unwired: 2 in, 2 out]
            n244 = property on="Wait unit" class="Str"("Visible"=w357) -> ()  [unwired: 2 in, 2 out]
          }
          frame True {
            w368 = u8 2 ("Disabled")
            n245 = property on="Units Tab" class="TabCtl (strict)"("Visible"=w367) -> ()  [unwired: 2 in, 2 out]
            n246 = property on="Dialog" class="Bool (strict)"("Disabled"=w368) -> ()  [unwired: 2 in, 2 out]
            n247 = Not(x=w367) -> (.not. x?=w366:bool)
            n248 = property on="Timeout" class="DigNum (strict)"("Visible"=w366) -> ()  [unwired: 2 in, 2 out]
            n249 = property on="Wait" class="Bool (strict)"("Disabled"=w368) -> ()  [unwired: 2 in, 2 out]
            n250 = property on="Dlg Def Val" class="Slide (strict)"("Visible"=w366) -> ()  [unwired: 2 in, 2 out]
            n251 = local read "Default Value"() -> (w363:dbl)
            n252 = property on="Wait unit" class="Str"("Visible"=w366) -> ()  [unwired: 2 in, 2 out]
            n253 = Greater Or Equal?(x=w363, y=0.01) -> (x >= y?=w364:bool)
            n254 = Select(t=w363, s=w364, f=0.0) -> (s? t:f=w361:dbl)
            n255 = local write "Default Value"(w361) -> ()
          }
        }
        n256 = local read "Interface Type"() -> (w353:u16)
        n257 = local read "GPIB Function"() -> (w354:u16)
        n258 = local read "RS-232 Func"() -> (w352:u16)
        n259 = local read "Operation"() -> (w351:i32)
        n260 = local read "Dialog"() -> (w350:bool)
        n261 = local read "Type"() -> (w355:u16)
        n262 = call "CRYMsgs Curves Gen Construct.vi"("Interface type"=w353, "GPIB func"=w354, "Step name"=w346, "Type"=w355, "RS232 func"=w352, "Operation"=w351, "Numeric?"=w349, "Dialog?"=w350) -> ("Curves generated"=w348:string[])  [unwired: 3 in]
        n263 = local read "Message Cluster"() -> (w356:T1)
        n264 = Bundle By Name(cluster=w356, "Numeric?"=w349, "Curves generated"=w348) -> (w347:T1)
        n265 = local write "Message Cluster"(w347) -> ()
      }
      event "Wait": Value Change {
        n266 = event-data() -> ("NewVal"=w370:bool)  [unwired: 6 out]
        n267 = local read "Message Cluster"() -> (w371:T1)
        n268 = case shown="True" w370 {
          frame False {
            w372 = FALSE ("Visible")
            n269 = property on="Timeout" class="DigNum (strict)"("Visible"=w372) -> ()  [unwired: 2 in, 2 out]
            n270 = property on="Wait unit" class="Str"("Visible"=w372) -> ()  [unwired: 2 in, 2 out]
          }
          frame True {
            n271 = property on="Timeout" class="DigNum (strict)"() -> ("Visible"=w380:bool)  [unwired: 2 in, 2 out]
            n272 = property on="No." class="Ring (strict)"() -> ("RingText.Text"=w377:string)  [unwired: 2 in, 2 out]
            n273 = local read "Type"() -> (w379:u16)
            n274 = case shown="False" w380 {
              frame False {
                w381 = TRUE ("Visible")
                n275 = property on="Timeout" class="DigNum (strict)"("Visible"=w381) -> ()  [unwired: 2 in, 2 out]
                n276 = property on="Wait unit" class="Str"("Visible"=w381) -> ()  [unwired: 2 in, 2 out]
              }
              frame True {
              }
            }
            n277 = Empty String/Path?(string/path=w377) -> (empty?=w375:bool)
            n278 = Equal?(x=w379, y=u16 2) -> (x = y?=w376:bool)
            n279 = Not(x=w375) -> (.not. x?=w374:bool)
            n280 = And(x=w376, y=w374) -> (x .and. y?=w373:bool)
            n281 = property on="Timeout" class="DigNum (strict)"("Caption.Visible"=w373) -> ()  [unwired: 2 in, 2 out]
          }
        }
        n282 = Bundle By Name(cluster=w371, "Wait?"=w370) -> (w369:T1)
        n283 = local write "Message Cluster"(w369) -> ()
      }
      event "Dialog": Value Change {
        n284 = event-data() -> ("NewVal"=w387:bool)  [unwired: 6 out]
        n285 = case shown="True" w387 {
          selector: w387 -> [w394 w400]
          frame False {
            w396 = u8 0 ("Disabled")
            n286 = Not(x=w394) -> (.not. x?=w397:bool)
            n287 = property on="Numeric" class="Bool (strict)"("Disabled"=w396, "Value"=FALSE ("Numeric")) -> ()  [unwired: 2 in, 2 out]
            n288 = property on="Flags" class="Slide (strict)"("Visible"=w397) -> ()  [unwired: 2 in, 2 out]
            n289 = property on="Dlg Def Val" class="Slide (strict)"("Visible"=w394) -> ()  [unwired: 2 in, 2 out]
            n290 = property on="Wait" class="Bool (strict)"("Disabled"=w396) -> ("Value"=w393:bool)  [unwired: 2 in, 2 out]
            n291 = property on="Units Tab" class="TabCtl (strict)"("Visible"=w394) -> ()  [unwired: 2 in, 2 out]
            n292 = property on="Timeout" class="DigNum (strict)"("Visible"=w393) -> ()  [unwired: 2 in, 2 out]
            n293 = property on="Wait unit" class="Str"("Visible"=w393) -> ()  [unwired: 2 in, 2 out]
          }
          frame True {
            w401 = u8 2 ("Disabled")
            n294 = Not(x=w400) -> (.not. x?=w399:bool)
            n295 = property on="Dlg Def Val" class="Slide (strict)"("Visible"=w400) -> ()  [unwired: 2 in, 2 out]
            n296 = property on="Numeric" class="Bool (strict)"("Disabled"=w401) -> ()  [unwired: 2 in, 2 out]
            n297 = property on="Flags" class="Slide (strict)"("Visible"=w399) -> ()  [unwired: 2 in, 2 out]
            n298 = Not(x=w400) -> (.not. x?=w398:bool)
            n299 = property on="Units Tab" class="TabCtl (strict)"("Visible"=w399) -> ()  [unwired: 2 in, 2 out]
            n300 = property on="Wait" class="Bool (strict)"("Disabled"=w401) -> ()  [unwired: 2 in, 2 out]
            n301 = property on="Timeout" class="DigNum (strict)"("Visible"=w398) -> ()  [unwired: 2 in, 2 out]
            n302 = property on="Wait unit" class="Str"("Visible"=w398) -> ()  [unwired: 2 in, 2 out]
          }
        }
        n303 = local read "Interface Type"() -> (w391:u16)
        n304 = local read "GPIB Function"() -> (w386:u16)
        n305 = local read "RS-232 Func"() -> (w390:u16)
        n306 = local read "Operation"() -> (w389:i32)
        n307 = local read "Numeric"() -> (w388:bool)
        n308 = local read "Type"() -> (w385:u16)
        n309 = call "CRYMsgs Curves Gen Construct.vi"("Interface type"=w391, "GPIB func"=w386, "Step name"=w382, "Type"=w385, "RS232 func"=w390, "Operation"=w389, "Numeric?"=w388, "Dialog?"=w387) -> ("Curves generated"=w384:string[])  [unwired: 3 in]
        n310 = local read "Message Cluster"() -> (w392:T1)
        n311 = Bundle By Name(cluster=w392, "Dialog?"=w387, "Curves generated"=w384) -> (w383:T1)
        n312 = local write "Message Cluster"(w383) -> ()
      }
      event "Operation": Value Change {
        n313 = event-data() -> ("NewVal"=w404:i32)  [unwired: 6 out]
        n314 = local read "GPIB Function"() -> (w412:u16)
        n315 = property on="Interface Type" class="Ring (strict)"() -> ("Value"=w414:u16)  [unwired: 2 in, 2 out]
        n316 = Equal To 0?(x=w414) -> (x = 0?=w413:bool)
        n317 = case shown="True" w413 {
          selector: w413 -> [_ w433]
          tunnel: w404 -> [w416 _]
          tunnel: w412 -> [w417 _]
          frame True {
            n318 = case shown="0, Default" w417 {
              tunnel: w416 -> [w420 _ _ _]
              frame 0, Default {
                w418 = FALSE
                w419 = TRUE ("Visible")
                n319 = case shown="1" w420 {
                  frame 0, Default {
                    w422 = FALSE ("Visible")
                    # "Read"
                    n320 = property on="Msg. term." class="Ring (strict)"("Visible"=w422) -> ()  [unwired: 2 in, 2 out]
                    n321 = property on="Timeout" class="DigNum (strict)"("Caption.Visible"=TRUE) -> ()  [unwired: 2 in, 2 out]
                    n322 = property on="Wait" class="Bool (strict)"("Visible"=w422) -> ()  [unwired: 2 in, 2 out]
                  }
                  frame 1 {
                    n323 = stacked-sequence {
                      frame #0 {
                        w423 = TRUE ("Visible")
                        # "Write"
                        n324 = property on="Msg. term." class="Ring (strict)"("Visible"=w423) -> ()  [unwired: 2 in, 2 out]
                        n325 = property on="Wait" class="Bool (strict)"("Visible"=w423) -> ()  [unwired: 2 in, 2 out]
                      }
                      frame #1 {
                        n326 = local read "Wait"() -> (w424:bool)
                        n327 = property on="Wait" class="Bool (strict)"("Val(Sgnl)"=w424) -> ()  [unwired: 2 in, 2 out]
                      }
                    }
                  }
                }
                n328 = property on="Operation" class="Slide (strict)"("Visible"=w419) -> ()  [unwired: 2 in, 2 out]
                n329 = property on="Command" class="Ring (strict)"("Visible"=w418) -> ()  [unwired: 2 in, 2 out]
                n330 = property on="Bytes" class="DigNum (strict)"("Visible"=w419) -> ()  [unwired: 2 in, 2 out]
                n331 = property on="Remote Enable" class="Bool (strict)"("Visible"=w418) -> ()  [unwired: 2 in, 2 out]
                n332 = property on="Command Msg" class="Str"("Visible"=w419) -> ()  [unwired: 2 in, 2 out]
              }
              frame 1 {
                n333 = stacked-sequence {
                  frame #0 {
                    w426 = FALSE
                    w425 = TRUE ("Visible")
                    n334 = property on="Command" class="Ring (strict)"("Visible"=w425) -> ()  [unwired: 2 in, 2 out]
                    n335 = property on="Command Msg" class="Str"("Visible"=w426) -> ()  [unwired: 2 in, 2 out]
                    n336 = property on="Operation" class="Slide (strict)"("Visible"=w426) -> ()  [unwired: 2 in, 2 out]
                    n337 = property on="Remote Enable" class="Bool (strict)"("Visible"=w425) -> ()  [unwired: 2 in, 2 out]
                    n338 = property on="Bytes" class="DigNum (strict)"("Visible"=w426) -> ()  [unwired: 2 in, 2 out]
                    n339 = property on="Msg. term." class="Ring (strict)"("Visible"=w426) -> ()  [unwired: 2 in, 2 out]
                    n340 = property on="Wait" class="Bool (strict)"("Visible"=w425) -> ()  [unwired: 2 in, 2 out]
                  }
                  frame #1 {
                    n341 = local read "Wait"() -> (w427:bool)
                    n342 = property on="Wait" class="Bool (strict)"("Val(Sgnl)"=w427) -> ()  [unwired: 2 in, 2 out]
                  }
                }
              }
              frame 2 {
                n343 = stacked-sequence {
                  frame #0 {
                    w428 = FALSE ("Visible")
                    n344 = property on="Command Msg" class="Str"("Visible"=w428) -> ()  [unwired: 2 in, 2 out]
                    n345 = property on="Command" class="Ring (strict)"("Visible"=w428) -> ()  [unwired: 2 in, 2 out]
                    n346 = property on="Wait" class="Bool (strict)"("Visible"=TRUE) -> ()  [unwired: 2 in, 2 out]
                    n347 = property on="Remote Enable" class="Bool (strict)"("Visible"=w428) -> ()  [unwired: 2 in, 2 out]
                    n348 = property on="Bytes" class="DigNum (strict)"("Visible"=w428) -> ()  [unwired: 2 in, 2 out]
                    n349 = property on="Msg. term." class="Ring (strict)"("Visible"=w428) -> ()  [unwired: 2 in, 2 out]
                    n350 = property on="Operation" class="Slide (strict)"("Visible"=w428) -> ()  [unwired: 2 in, 2 out]
                  }
                  frame #1 {
                    n351 = local read "Wait"() -> (w430:bool)
                    n352 = property on="Wait" class="Bool (strict)"("Val(Sgnl)"=w430) -> ()  [unwired: 2 in, 2 out]
                  }
                }
              }
              frame 3 {
                w431 = TRUE ("Visible")
                w432 = FALSE ("Visible")
                n353 = property on="Command Msg" class="Str"("Visible"=w432) -> ()  [unwired: 2 in, 2 out]
                n354 = property on="Operation" class="Slide (strict)"("Visible"=w432) -> ()  [unwired: 2 in, 2 out]
                n355 = property on="Command" class="Ring (strict)"("Visible"=w432) -> ()  [unwired: 2 in, 2 out]
                n356 = property on="Timeout" class="DigNum (strict)"("Visible"=w431, "Caption.Visible"=w431) -> ()  [unwired: 2 in, 2 out]
                n357 = property on="Msg. term." class="Ring (strict)"("Visible"=w432) -> ()  [unwired: 2 in, 2 out]
                n358 = property on="Remote Enable" class="Bool (strict)"("Visible"=w432) -> ()  [unwired: 2 in, 2 out]
                n359 = property on="Bytes" class="DigNum (strict)"("Visible"=w432) -> ()  [unwired: 2 in, 2 out]
                n360 = property on="Wait unit" class="Str"("Visible"=w431) -> ()  [unwired: 2 in, 2 out]
                n361 = property on="Wait" class="Bool (strict)"("Visible"=w432) -> ()  [unwired: 2 in, 2 out]
              }
            }
          }
          frame False {
            w434 = TRUE ("Visible")
            n362 = Not(x=w433) -> (.not. x?=w435:bool)
            n363 = property on="Timeout" class="DigNum (strict)"("Visible"=w434, "Caption.Visible"=w434) -> ()  [unwired: 2 in, 2 out]
            n364 = property on="Wait" class="Bool (strict)"("Visible"=w435, "Value"=w435) -> ()  [unwired: 2 in, 2 out]
          }
        }
        n365 = local read "Interface Type"() -> (w409:u16)
        n366 = local read "GPIB Function"() -> (w410:u16)
        n367 = local read "RS-232 Func"() -> (w408:u16)
        n368 = local read "Numeric"() -> (w406:bool)
        n369 = local read "Dialog"() -> (w407:bool)
        n370 = local read "Type"() -> (w411:u16)
        n371 = call "CRYMsgs Curves Gen Construct.vi"("Interface type"=w409, "GPIB func"=w410, "Step name"=w402, "Type"=w411, "RS232 func"=w408, "Operation"=w404, "Numeric?"=w406, "Dialog?"=w407) -> ("Curves generated"=w405:string[])  [unwired: 3 in]
        n372 = local read "Message Cluster"() -> (w415:T1)
        n373 = Bundle By Name(cluster=w415, "Operation"=w404, "Curves generated"=w405) -> (w403:T1)
        n374 = local write "Message Cluster"(w403) -> ()
      }
      event "Message Title": Value Change {
        n375 = event-data() -> ("NewVal"=w437:string)  [unwired: 6 out]
        n376 = local read "Message Cluster"() -> (w438:T1)
        n377 = Bundle By Name(cluster=w438, "Message Tilte"=w437) -> (w436:T1)
        n378 = local write "Message Cluster"(w436) -> ()
      }
      event "Command Msg": Value Change {
        n379 = event-data() -> ("NewVal"=w440:string)  [unwired: 6 out]
        n380 = local read "Message Cluster"() -> (w441:T1)
        n381 = Bundle By Name(cluster=w441, "Command Msg"=w440) -> (w439:T1)
        n382 = local write "Message Cluster"(w439) -> ()
      }
      event "Timeout": Value Change {
        n383 = event-data() -> ("NewVal"=w443:i32)  [unwired: 6 out]
        n384 = local read "Message Cluster"() -> (w444:T1)
        n385 = Bundle By Name(cluster=w444, "Pause [ms]"=w443) -> (w442:T1)
        n386 = local write "Message Cluster"(w442) -> ()
      }
      event "Units": Value Change {
        n387 = event-data() -> ("NewVal"=w447:string)  [unwired: 6 out]
        n388 = local read "Message Cluster"() -> (w446:T1)
        n389 = Bundle By Name(cluster=w446, "Print Unit"=w447) -> (w445:T1)
        n390 = local write "Message Cluster"(w445) -> ()
      }
      event "Units Cluster": Value Change {
        n391 = event-data() -> ("NewVal"=w449:T5)  [unwired: 6 out]
        n392 = local read "Message Cluster"() -> (w450:T1)
        n393 = Bundle By Name(cluster=w450, "Units"=w449) -> (w448:T1)
        n394 = local write "Message Cluster"(w448) -> ()
      }
      event "Default Value": Value Change {
        n395 = event-data() -> ("NewVal"=w452:dbl)  [unwired: 6 out]
        n396 = local read "Message Cluster"() -> (w453:T1)
        n397 = Bundle By Name(cluster=w453, "Default Value"=w452) -> (w451:T1)
        n398 = local write "Message Cluster"(w451) -> ()
      }
      event "Axis": Value Change {
        n399 = event-data() -> ("NewVal"=w455:u16)  [unwired: 6 out]
        n400 = local read "Message Cluster"() -> (w456:T1)
        n401 = Bundle By Name(cluster=w456, "Axis"=w455) -> (w454:T1)
        n402 = local write "Message Cluster"(w454) -> ()
      }
      event "Dlg Def Val": Value Change {
        n403 = event-data() -> ("NewVal"=w459:u16)  [unwired: 6 out]
        n404 = disable-structure shown="Disabled" {
          disable-tunnel: _ -> [w461 _]
          frame Disabled {
            # "Same as Default"
            n405 = local read "Message Cluster"() -> (w462:T1)
            n406 = Bundle By Name(cluster=w462, "Default Value"=w461) -> (w460:T1)
            n407 = local write "Message Cluster"(w460) -> ()
          }
          frame Enabled {
          }
        }
        n408 = local read "Message Cluster"() -> (w458:T1)
        n409 = Bundle By Name(cluster=w458, "Default Value"=w459) -> (w457:T1)
        n410 = local write "Message Cluster"(w457) -> ()
      }
      event Value Change {
        n411 = event-data() -> ("NewVal"=w464:T4)  [unwired: 6 out]
        n412 = local read "Message Cluster"() -> (w465:T1)
        n413 = Bundle By Name(cluster=w465, "Text Format"=w464) -> (w463:T1)
        n414 = local write "Message Cluster"(w463) -> ()
      }
      event "Port": Value Change {
        n415 = event-data() -> ("NewVal"=w466:i32)  [unwired: 6 out]
        n416 = local read "DIO Array"() -> (w468:bool[])
        n417 = Index Array(array=w468, index=w466) -> (element=w467:bool)
        n418 = property on="DIO Array" class="Arr (strict)"() -> ("Value"=w471:bool[])  [unwired: 2 in, 2 out]
        n419 = local read "Message Cluster"() -> (w472:T1)
        n420 = local write "DIO direction"(w467) -> ()
        n421 = Index Array(array=w471, index=w466) -> (element=w470:bool)
        n422 = Bundle By Name(cluster=w472, "Port #"=w466) -> (w469:T1)
        n423 = property on="DIO direction" class="Bool (strict)"("Value"=w470) -> ()  [unwired: 2 in, 2 out]
        n424 = local write "Message Cluster"(w469) -> ()
      }
      event "Line selected": Value Change {
        n425 = event-data() -> ("NewVal"=w474:T2)  [unwired: 6 out]
        n426 = Cluster To Array(cluster=w474) -> (array=w478:bool[])
        n427 = Boolean Array To Number(Boolean array=w478) -> (number=w477:u32)
        n428 = local read "Message Cluster"() -> (w476:T1)
        n429 = To Unsigned Long Integer(number=w477) -> (unsigned 32bit integer=w475:u32)
        n430 = Bundle By Name(cluster=w476, "Line selected"=w475) -> (w473:T1)
        n431 = local write "Message Cluster"(w473) -> ()
      }
      event "Line selected 2": Value Change {
        n432 = event-data() -> ("NewVal"=w480:T2)  [unwired: 6 out]
        n433 = Cluster To Array(cluster=w480) -> (array=w484:bool[])
        n434 = Boolean Array To Number(Boolean array=w484) -> (number=w483:u32)
        n435 = local read "Message Cluster"() -> (w482:T1)
        n436 = To Unsigned Long Integer(number=w483) -> (unsigned 32bit integer=w481:u32)
        n437 = Bundle By Name(cluster=w482, "Line selected 2"=w481) -> (w479:T1)
        n438 = local write "Message Cluster"(w479) -> ()
      }
      event "Pattern": Value Change {
        n439 = event-data() -> ("NewVal"=w486:T3)  [unwired: 6 out]
        n440 = Cluster To Array(cluster=w486) -> (array=w490:bool[])
        n441 = Boolean Array To Number(Boolean array=w490) -> (number=w489:u32)
        n442 = local read "Message Cluster"() -> (w488:T1)
        n443 = To Unsigned Long Integer(number=w489) -> (unsigned 32bit integer=w487:u32)
        n444 = Bundle By Name(cluster=w488, "pattern"=w487) -> (w485:T1)
        n445 = local write "Message Cluster"(w485) -> ()
      }
      event "Pattern 2": Value Change {
        n446 = event-data() -> ("NewVal"=w492:T3)  [unwired: 6 out]
        n447 = Cluster To Array(cluster=w492) -> (array=w496:bool[])
        n448 = Boolean Array To Number(Boolean array=w496) -> (number=w495:u32)
        n449 = local read "Message Cluster"() -> (w494:T1)
        n450 = To Unsigned Long Integer(number=w495) -> (unsigned 32bit integer=w493:u32)
        n451 = Bundle By Name(cluster=w494, "pattern 2"=w493) -> (w491:T1)
        n452 = local write "Message Cluster"(w491) -> ()
      }
      event "No.": Value Change {
        n453 = event-data() -> ("NewVal"=w509:u8)  [unwired: 6 out]
        n454 = property on="Interface Name" class="Arr (strict)"() -> ("Value"=w507:u16[])  [unwired: 2 in, 2 out]
        n455 = Index Array(array=w507, index=w509) -> (element=w498:u16)
        n456 = local read "GPIB Function"() -> (w505:u16)
        n457 = local read "RS-232 Func"() -> (w504:u16)
        n458 = local write "Interface Type"(w498) -> ()
        n459 = local read "Operation"() -> (w503:i32)
        n460 = local read "Numeric"() -> (w501:bool)
        n461 = local read "Dialog"() -> (w502:bool)
        n462 = local read "Type"() -> (w506:u16)
        n463 = call "CRYMsgs Curves Gen Construct.vi"("Interface type"=w498, "GPIB func"=w505, "Step name"=w497, "Type"=w506, "RS232 func"=w504, "Operation"=w503, "Numeric?"=w501, "Dialog?"=w502) -> ("Curves generated"=w500:string[])  [unwired: 3 in]
        n464 = case shown="1..3, Default" w498 {
          selector: w498 -> [_ w514]
          frame 0 {
            w511 = TRUE ("Visible")
            w510 = FALSE ("Visible")
            # "IEEE488"
            n465 = property on="GPIB Function" class="Ring (strict)"("Visible"=w511) -> ()  [unwired: 2 in, 2 out]
            n466 = property on="GPIB Function" class="Ring (strict)"() -> ("Value"=w512:u16)  [unwired: 2 in, 2 out]
            n467 = property on="RS-232 Func" class="Ring (strict)"("Visible"=w510) -> ()  [unwired: 2 in, 2 out]
            n468 = property on="Format Text" class="Bool (strict)"("Visible"=w510) -> ()  [unwired: 2 in, 2 out]
            n469 = property on="Serial Ctrl line Read" class="Slide (strict)"("Visible"=w510) -> ()  [unwired: 2 in, 2 out]
            n470 = property on="Address" class="DigNum (strict)"("Visible"=w511) -> ()  [unwired: 2 in, 2 out]
            n471 = property on="GPIB Function" class="Ring (strict)"("Val(Sgnl)"=w512) -> ()  [unwired: 2 in, 2 out]
            n472 = property on="Serial Ctrl line" class="Slide (strict)"("Visible"=w510) -> ()  [unwired: 2 in, 2 out]
          }
          frame 1..3, Default {
            w515 = u16 0 items=["IEEE-488", "RS-232", "Footswitch", "Buzzer"] ("Interface Type")
            w516 = FALSE
            # "RS232 & others"
            n473 = Not Equal?(x=w514, y=w515) -> (x != y?=w513:bool)
            n474 = case shown="True" w513 {
              frame True {
                n475 = property on="RS-232 Func" class="Ring (strict)"() -> ("Value"=w519:u16)  [unwired: 2 in, 2 out]
                n476 = property on="RS-232 Func" class="Ring (strict)"("Visible"=TRUE) -> ()  [unwired: 2 in, 2 out]
                n477 = property on="GPIB Function" class="Ring (strict)"("Visible"=FALSE) -> ()  [unwired: 2 in, 2 out]
                n478 = property on="RS-232 Func" class="Ring (strict)"("Val(Sgnl)"=w519) -> ()  [unwired: 2 in, 2 out]
              }
              frame False {
                n479 = property on="RS-232 Func" class="Ring (strict)"("Visible"=FALSE) -> ()  [unwired: 2 in, 2 out]
                n480 = property on="GPIB Function" class="Ring (strict)"("Visible"=TRUE) -> ()  [unwired: 2 in, 2 out]
              }
            }
            n481 = property on="Msg. term." class="Ring (strict)"("Visible"=w516) -> ()  [unwired: 2 in, 2 out]
            n482 = property on="Command" class="Ring (strict)"("Visible"=w516) -> ()  [unwired: 2 in, 2 out]
            n483 = property on="Address" class="DigNum (strict)"("Visible"=w516) -> ()  [unwired: 2 in, 2 out]
            n484 = property on="Format Text" class="Bool (strict)"("Visible"=w516) -> ()  [unwired: 2 in, 2 out]
            n485 = property on="Remote Enable" class="Bool (strict)"("Visible"=w516) -> ()  [unwired: 2 in, 2 out]
            n486 = property on="Bytes" class="DigNum (strict)"("Visible"=w516) -> ()  [unwired: 2 in, 2 out]
          }
        }
        n487 = local read "Message Cluster"() -> (w508:T1)
        n488 = Bundle By Name(cluster=w508, "Curves generated"=w500, "Interf #"=w509) -> (w499:T1)
        n489 = local write "Message Cluster"(w499) -> ()
      }
      event "Address": Value Change {
        n490 = event-data() -> ("NewVal"=w524:i32)  [unwired: 6 out]
        n491 = Number To Decimal String(number=w524) -> (decimal integer string=w523:string)  [unwired: 1 out]
        n492 = local read "Message Cluster"() -> (w525:T1)
        n493 = Bundle By Name(cluster=w525, "Address"=w523) -> (w522:T1)
        n494 = local write "Message Cluster"(w522) -> ()
      }
      event "Msg. term.": Value Change {
        n495 = event-data() -> ("NewVal"=w527:i32)  [unwired: 6 out]
        n496 = local read "Message Cluster"() -> (w528:T1)
        n497 = Bundle By Name(cluster=w528, "GPIB term"=w527) -> (w526:T1)
        n498 = local write "Message Cluster"(w526) -> ()
      }
      event "Bytes": Value Change {
        n499 = event-data() -> ("NewVal"=w530:i32)  [unwired: 6 out]
        n500 = local read "Message Cluster"() -> (w531:T1)
        n501 = Bundle By Name(cluster=w531, "bytes"=w530) -> (w529:T1)
        n502 = local write "Message Cluster"(w529) -> ()
      }
      event "Command": Value Change {
        n503 = event-data() -> ("NewVal"=w533:u16)  [unwired: 6 out]
        n504 = local read "Message Cluster"() -> (w534:T1)
        n505 = Bundle By Name(cluster=w534, "GPIB cmd"=w533) -> (w532:T1)
        n506 = local write "Message Cluster"(w532) -> ()
      }
      event "Remote Enable": Value Change {
        n507 = event-data() -> ("NewVal"=w536:bool)  [unwired: 6 out]
        n508 = local read "Message Cluster"() -> (w537:T1)
        n509 = Bundle By Name(cluster=w537, "GPIB rem en"=w536) -> (w535:T1)
        n510 = local write "Message Cluster"(w535) -> ()
      }
      event "Help": Value Change {
        n511 = event-data() -> ("NewVal"=w539:string)  [unwired: 6 out]
        n512 = local read "Message Cluster"() -> (w540:T1)
        n513 = Bundle By Name(cluster=w540, "Help"=w539) -> (w538:T1)
        n514 = local write "Message Cluster"(w538) -> ()
      }
      event "Main Tab": Value Change {
        n515 = event-data() -> ("NewVal"=w542:enum32{"Setting", "Help"})  [unwired: 6 out]
        n516 = local read "Message Cluster"() -> (w543:T1)
        n517 = Bundle By Name(cluster=w543, "Tab Value"=w542) -> (w541:T1)
        n518 = local write "Message Cluster"(w541) -> ()
      }
      event "Serial Ctrl line": Value Change {
        n519 = event-data() -> ()  [unwired: 7 out]
        n520 = local read "Serial Ctrl line Read"() -> (w547:u16)
        n521 = local read "RS-232 Func"() -> (w549:u16)
        n522 = local read "Serial Ctrl line"() -> (w548:u16)
        n523 = case shown="2" w549 {
          tunnel: w548 -> [w550 _]
          tunnel: w547 -> [_ w551]
          tunnel: [w550 w551] -> w545
          frame Default {
          }
          frame 2 {
          }
        }
        n524 = local read "Message Cluster"() -> (w546:T1)
        n525 = Bundle By Name(cluster=w546, "Serial Ctrl lines"=w545) -> (w544:T1)
        n526 = local write "Message Cluster"(w544) -> ()
      }
      event "Serial Ctrl line Read": Value Change {
        n527 = event-data() -> ()  [unwired: 7 out]
        n528 = local read "Serial Ctrl line Read"() -> (w555:u16)
        n529 = local read "RS-232 Func"() -> (w557:u16)
        n530 = local read "Serial Ctrl line"() -> (w556:u16)
        n531 = case shown="Default" w557 {
          tunnel: w556 -> [w558 _]
          tunnel: w555 -> [_ w559]
          tunnel: [w558 w559] -> w553
          frame Default {
          }
          frame 2 {
          }
        }
        n532 = local read "Message Cluster"() -> (w554:T1)
        n533 = Bundle By Name(cluster=w554, "Serial Ctrl lines"=w553) -> (w552:T1)
        n534 = local write "Message Cluster"(w552) -> ()
      }
      event "Digital IO Update": Value Change {
        n535 = event-data() -> ()  [unwired: 7 out]
        n536 = flat-sequence {
          tunnel: w560 -> [w571]
          frame #0 {
            n537 = local read "Message Cluster"() -> (w570:T1)
            n538 = Unbundle By Name(w570) -> ("G_Bits"=w577:T14, "H_Bits"=w576:T14)
            n539 = local read "Line selected 2"() -> (w573:T2)
            n540 = local read "Line selected"() -> (w575:T2)
            n541 = local read "Pattern 2"() -> (w572:T3)
            n542 = local read "Pattern"() -> (w574:T3)
            n543 = call "CRYDigital IO Update.vi"("No.VI"=w571, "Pattern"=w572, "Line selected"=w573, "Bits Cluster"=w576) -> ("Pattern Out"=w563:T3)  [unwired: 7 in]
            n544 = call "CRYDigital IO Update.vi"("No.VI"=w571, "Pattern"=w574, "Line selected"=w575, "Bits Cluster"=w577) -> ("Pattern Out"=w562:T3)  [unwired: 7 in]
            n545 = local write "Pattern"(w562) -> ()
            n546 = local write "Pattern 2"(w563) -> ()
            n547 = Cluster To Array(cluster=w563) -> (array=w565:bool[])
            n548 = Cluster To Array(cluster=w562) -> (array=w569:bool[])
            n549 = Boolean Array To Number(Boolean array=w565) -> (number=w566:u32)
            n550 = Boolean Array To Number(Boolean array=w569) -> (number=w568:u32)
            n551 = To Unsigned Long Integer(number=w566) -> (unsigned 32bit integer=w564:u32)
            n552 = To Unsigned Long Integer(number=w568) -> (unsigned 32bit integer=w561:u32)
            n553 = Bundle By Name(cluster=w570, "pattern"=w561, "pattern 2"=w564) -> (w567:T1)
            n554 = local write "Message Cluster"(w567) -> ()
          }
          frame #1 {
          }
        }
      }
    }
    n555 = global read "CRYMain Sub Window Global.vi" "gStop"() -> (w53:bool)
    n556 = Or(x=w53, y="stop") -> (x .or. y?=w52:bool)
    n557 = Bundle("Load Test"="Load Test", "Format Text"="Format Text", "Unit Control"="Unit Control", "Apply"="Apply", "Add Lib"="Add Lib", "OK"="OK", "Cancel"="Cancel", "Setting"="Setting") -> (w60:T15)  [unwired: 1 out]
    n558 = Cluster To Array(cluster=w60) -> (array=w61:bool[])
    n559 = Search 1D Array(1D array=w61, element=TRUE) -> (index of element=w58:i32)  [unwired: 1 out]
    n560 = case shown="4" w58 {
      tunnel: w48 -> [_ _ _ _ w146 _ _ _ _]
      tunnel: w42 -> [_ _ _ _ _ w162 _ _ w200]
      frame Default {
      }
      frame 0 {
        n561 = stacked-sequence {
          seq-local: [w62 _ _ _ _ _] -> [_ _ _ _ _ w112]
          frame #0 {
            n562 = local read "Message Cluster"() -> (w101:T1)
            n563 = Unbundle By Name(w101) -> ("Type"=w62:u16, "Message Tilte"=w94:string, "Flags"=w93:u16, "Wait?"=w92:bool, "Numeric?"=w91:bool, "Dialog?"=w90:bool, "Pause [ms]"=w89:i32, "pattern"=w98:u32, "Line selected"=w97:u32, "Address"=w96:string, "Operation"=w85:i32, "bytes"=w84:i32, "Command Msg"=w83:string, "RS232 Func"=w71:u16, "Serial Ctrl lines"=w70:u16, "Interf #"=w82:u8, "GPIB func"=w81:u16, "GPIB cmd"=w80:u16, "GPIB rem en"=w79:bool, "GPIB term"=w78:i32, "Print Unit"=w77:string, "Axis"=w76:u16, "Default Value"=w75:dbl, "Port #"=w69:i32, "Units"=w74:T5, "Text Format"=w95:T16, "Help"=w73:string, "Tab Value"=w72:enum32{"Setting", "Help"}, "pattern 2"=w66:u32, "Line selected 2"=w65:u32)  [unwired: 1 out]
            n564 = Number To Boolean Array(number=w98) -> (Boolean array=w99:bool[])
            n565 = Number To Boolean Array(number=w65) -> (Boolean array=w67:bool[])
            n566 = Number To Boolean Array(number=w66) -> (Boolean array=w68:bool[])
            n567 = Array To Cluster(array=w99) -> (cluster=w88:T17)
            n568 = Number To Boolean Array(number=w97) -> (Boolean array=w100:bool[])
            n569 = local write "Dlg Def Val"(w75) -> ()
            n570 = Array To Cluster(array=w67) -> (cluster=w63:T17)
            n571 = Array To Cluster(array=w68) -> (cluster=w64:T17)
            n572 = Array To Cluster(array=w100) -> (cluster=w87:T17)
            n573 = property on="Help" class="Str"("Value"=w73) -> ()  [unwired: 2 in, 2 out]
            n574 = local write "Command Msg"(w83) -> ()
            n575 = local write "Command"(w80) -> ()
            n576 = local write "Message Title"(w94) -> ()
            n577 = local write "Numeric"(w91) -> ()
            n578 = local write "GPIB Function"(w81) -> ()
            n579 = local write "Units Cluster"(w74) -> ()
            n580 = local write "Dialog"(w90) -> ()
            n581 = local write "Timeout"(w89) -> ()
            n582 = local write "Line selected"(w87) -> ()
            n583 = local write "Remote Enable"(w79) -> ()
            n584 = local write "Default Value"(w75) -> ()
            n585 = local write "Text Format"(w95) -> ()
            n586 = local write "Operation"(w85) -> ()
            n587 = local write "Msg. term."(w78) -> ()
            n588 = local write "Type"(w62) -> ()
            n589 = local write "Flags"(w93) -> ()
            n590 = local write "Wait"(w92) -> ()
            n591 = local write "Pattern"(w88) -> ()
            n592 = local write "Bytes"(w84) -> ()
            n593 = local write "No."(w82) -> ()
            n594 = local write "Units"(w77) -> ()
            n595 = local write "Axis"(w76) -> ()
            n596 = local write "Line selected 2"(w63) -> ()
            n597 = local write "Pattern 2"(w64) -> ()
            n598 = property on="Main Tab" class="TabCtl (strict)"("Value"=w72) -> ()  [unwired: 2 in, 2 out]
            n599 = property on="Port" class="Ring (strict)"("Val(Sgnl)"=w69) -> ()  [unwired: 2 in, 2 out]
            n600 = Decimal String To Number(string=w96) -> (number=w86:i32)  [unwired: 3 out]
            n601 = case shown="Default" w71 {
              tunnel: w70 -> [w102 w103]
              frame Default {
                n602 = local write "Serial Ctrl line"(w102) -> ()
              }
              frame 2 {
                n603 = local write "Serial Ctrl line Read"(w103) -> ()
              }
            }
            n604 = local write "RS-232 Func"(w71) -> ()
            n605 = local write "Address"(w86) -> ()
          }
          frame #1 {
            n606 = control-ref of="Board Tab"() -> (w104:refnum<vi>)
            n607 = control-ref of="This VI"() -> (w106:refnum<vi>)
            n608 = call "CRYAlign Steps VI Center.vi"("Tab2"=w104, "Input/Output"=TRUE, "VIRef"=w106) -> ()  [unwired: 1 in, 8 out]
          }
          frame #2 {
            n609 = property on="Board Tab" class="TabCtl (strict)"("Visible"=TRUE) -> ()  [unwired: 2 in, 2 out]
            n610 = property on="Load Test" class="Bool (strict)"("Value"=FALSE ("Load Test")) -> ()  [unwired: 2 in, 2 out]
          }
          frame #3 {
            n611 = local read "Type"() -> (w110:u16)
            n612 = property on="Digital IO Update" class="Bool (strict)"("Val(Sgnl)"=TRUE ("Value (Signaling)")) -> ()  [unwired: 2 in, 2 out]
            n613 = property on="Type" class="Slide (strict)"("Val(Sgnl)"=w110) -> ()  [unwired: 2 in, 2 out]
          }
          frame #4 {
            n614 = local read "AddStep"() -> (w111:bool)
            n615 = local write "Add Lib"(w111) -> ()
          }
          frame #5 {
            n616 = flat-sequence {
              tunnel: w112 -> [w114]
              frame #0 {
                n617 = local write "AddStep"(FALSE ("AddStep")) -> ()
              }
              frame #1 {
                n618 = case shown="1" w114 {
                  frame 0, Default {
                  }
                  frame 1 {
                    n619 = property on="Apply" class="Bool (strict)"("Value"=FALSE ("Apply")) -> ()  [unwired: 2 in, 2 out]
                  }
                }
              }
            }
          }
        }
      }
      frame 1 {
        n620 = property on="Command Msg" class="Str"() -> ("Value"=w118:string)  [unwired: 2 in, 2 out]
        n621 = call "CRYFormat Text.vi"("Text Format In"="Text Format", "Text In"=w118) -> ("Text Format Out"=w116:T4)  [unwired: 8 out]
        n622 = property on="Format Text" class="Bool (strict)"("Value"=FALSE ("Format Text")) -> ()  [unwired: 2 in, 2 out]
        n623 = property on="Text Format" class="Clust (strict)"("Val(Sgnl)"=w116) -> ()  [unwired: 2 in, 2 out]
      }
      frame 2 {
        n624 = Unbundle By Name("Units Cluster") -> ("axis"=w120:u16, "unit"=w131:string, "dB ref"=w130:dbl, "Common dB ref."=w121:u16)
        n625 = Bundle(FALSE, FALSE) -> (w134:cluster{bool, bool})  [unwired: 1 out]
        n626 = property on="Unit Control" class="Bool (strict)"("Value"=FALSE ("Unit...")) -> ()  [unwired: 2 in, 2 out]
        n627 = call "CRYUnits setup.vi"("Scale visible?"=TRUE, "dB/Lin"=w120, "Unit:"=w131, "dB ref:"=w130, "Custom unit settings"=w134, "Common dB ref."=w121) -> ("New Scale"=w123:u16, "New unit Lin"=w126:string, "New dB ref"=w129:dbl, "Common dB #"=w122:u16, "Cancelled?"=w124:bool, "Common dB"=w127:string)  [unwired: 2 in, 2 out]
        n628 = case shown="False" w124 {
          tunnel: w129 -> [_ w140]
          tunnel: w127 -> [_ w141]
          tunnel: w126 -> [_ w139]
          tunnel: "Units Cluster" -> [_ w143]
          tunnel: w123 -> [_ w137]
          tunnel: w122 -> [_ w136]
          frame True {
          }
          frame False {
            n629 = call "CRYGet Print Unit.vi"("dB ref"=w140, "Unit"=w139, "Common dB #"=w136, "Common dB"=w141, "Scale"=w137) -> ("Print Unit"=w138:string)  [unwired: 6 out]
            n630 = Bundle By Name(cluster=w143, "unit"=w139, "dB ref"=w140, "Common dB ref."=w136, "axis"=w137) -> (w142:T5)
            n631 = property on="Units" class="Str"("Val(Sgnl)"=w138) -> ()  [unwired: 2 in, 2 out]
            n632 = property on="Units Cluster" class="Clust (strict)"("Val(Sgnl)"=w142) -> ()  [unwired: 2 in, 2 out]
          }
        }
      }
      frame 3 {
        n633 = global read "CRYMainGlobal.vi" "Access Level"() -> (w145:enum16{"Engineer", "Technician", "Operator"})
        n634 = case shown="\"Operator\", Default" w145 {
          tunnel: w146 -> [w147 _]
          frame "Engineer" {
            n635 = flat-sequence {
              tunnel: [w149] -> w148
              tunnel: w147 -> [w153]
              tunnel: w148 -> [w156]
              frame #0 {
                n636 = call "CRYGet Current TS Steps.vi"() -> ("SelectStepNumber in Tree"=w151:i32, "Steps"=w150:T7[])  [unwired: 1 in, 9 out]
                n637 = Index Array(array=w150, index=w151) -> (element=w149:T7)
              }
              frame #1 {
                n638 = local read "Message Cluster"() -> (w152:T1)
                n639 = call "CRYFlatten Messages.vi"("Messages"=w152) -> ("Flatten Messages String"=w155:string)  [unwired: 10 out]
                n640 = Bundle By Name(cluster=w156, "Seq setup flattened"=w155) -> (w154:T7)
                n641 = call "CRYMessages.vi"("Setup in"=w154, "Step name"=w153) -> ()  [unwired: 7 in, 7 out]
              }
              frame #2 {
                n642 = property on="Apply" class="Bool (strict)"("Value"=FALSE ("Apply")) -> ()  [unwired: 2 in, 2 out]
              }
            }
          }
          frame "Operator", Default {
            n643 = call "CRYGet Error Message.vi"("Kind"="Step Setup") -> ("Window Title"=w159:string)  [unwired: 5 in, 5 out]
            n644 = call "CRYGet Access Level Message.vi"() -> ("Multibyte string"=w161:string)  [unwired: 11 in]
            n645 = call "CRYMessage Dialog.vi"("Window Title"=w159, "YesNoCancel"=T12."OK", "Message Content"=w161) -> ()  [unwired: 7 in, 2 out]
          }
        }
        n646 = local write "Apply"(FALSE ("Apply")) -> ()
      }
      frame 4 {
        n647 = flat-sequence {
          tunnel: w162 -> [w169]
          frame #0 {
            n648 = local read "Message Cluster"() -> (w163:T1)
            n649 = call "CRYGet Current TS Steps.vi"() -> ("SelectStepNumber in Tree"=w165:i32, "Steps"=w166:T7[])  [unwired: 7 in, 3 out]
            n650 = call "CRYFlatten Messages.vi"("Messages"=w163) -> ("Flatten Messages String"=w168:string)  [unwired: 10 in]
            n651 = Index Array(array=w166, index=w165) -> (element=w164:T7)
            n652 = call "CRYMessage Name Insert.vi"("Setup in"=w164, "Step setup in"=w168, "Type In"="AddStep") -> ()  [unwired: 9 in]
          }
          frame #1 {
            n653 = global read "CRYStepSetup Global.vi" "Load from AddStep"() -> (w170:bool)
            n654 = local write "Add Lib"(FALSE ("Add Lib")) -> ()
            n655 = case shown="True" w170 {
              tunnel: w169 -> [_ w173]
              frame False {
              }
              frame True {
                n656 = global write "CRYStepSetup Global.vi" "Load from AddStep"(FALSE ("Load from AddStep")) -> ()
                n657 = call "CRYStepData Manipulate.vi"("sAction"="Backup", "StepNo."=w173) -> ()  [unwired: 10 in]
              }
            }
          }
        }
      }
      frame 5 {
        n658 = flat-sequence {
          frame #0 {
            n659 = global read "CRYMainGlobal.vi" "Access Level"() -> (w176:enum16{"Engineer", "Technician", "Operator"})
            n660 = case shown="\"Technician\", Default" w176 {
              frame "Engineer" {
                n661 = flat-sequence {
                  tunnel: [w178] -> w177
                  tunnel: w177 -> [w184]
                  frame #0 {
                    n662 = local read "Message Cluster"() -> (w183:T1)
                    n663 = local read "Proper VI No"() -> (w179:i32)
                    n664 = call "CRYFlatten Messages.vi"("Messages"=w183) -> ("Flatten Messages String"=w178:string)  [unwired: 10 out]
                    n665 = call "CRYPreUpdate Sequence.vi"("EventName"="SequenceUpdate", "Proper VI No"=w179, "Project View Step Name Identifier Arg1"="", "Step flattened Arg2"=w178, "AllChangeFlg"=TRUE ("Name/Identifier")) -> ()  [unwired: 11 in]
                  }
                  frame #1 {
                    n666 = call "CRYGet Current TS Steps.vi"() -> ("SelectStepNumber in Tree"=w186:i32, "Steps"=w187:T7[])  [unwired: 7 in, 3 out]
                    n667 = Index Array(array=w187, index=w186) -> (element=w185:T7)
                    n668 = call "CRYMessage Name Insert.vi"("Setup in"=w185, "Step setup in"=w184, "Type In"="StepOK") -> ()  [unwired: 9 in]
                  }
                }
              }
              frame "Technician", Default {
                n669 = call "CRYGet Error Message.vi"("Kind"="Step Setup") -> ("Window Title"=w191:string)  [unwired: 5 in, 5 out]
                n670 = call "CRYGet Access Level Message.vi"("sAction"="OK") -> ("Multibyte string"=w193:string)  [unwired: 10 in]
                n671 = call "CRYMessage Dialog.vi"("Window Title"=w191, "YesNoCancel"=T12."OK", "Message Content"=w193) -> ()  [unwired: 7 in, 2 out]
              }
            }
          }
          frame #1 {
            n672 = local write "OK"(FALSE ("OK")) -> ()
          }
        }
        n673 = local write "stop"(TRUE ("stop")) -> ()
      }
      frame 6 {
        n674 = flat-sequence {
          frame #0 {
            n675 = local read "Proper VI No"() -> (w196:i32)
            n676 = call "CRYStepData Manipulate.vi"("sAction"="Restore", "StepNo."=w196) -> ()  [unwired: 10 in]
          }
          frame #1 {
            n677 = local write "Cancel"(FALSE ("Cancel")) -> ()
          }
        }
        n678 = local write "stop"(TRUE ("stop")) -> ()
      }
      frame 7 {
        n679 = flat-sequence {
          tunnel: w200 -> [w204]
          tunnel: [w203] -> w199
          tunnel: w199 -> [w206]
          frame #0 {
            n680 = local read "Message Cluster"() -> (w202:T1)
            n681 = call "CRYDigital IO Setting.vi"("No.VI"=w204, "Message Cluster"=w202) -> ("Result"=w203:bool, "Message Cluster Out"=w201:T1)  [unwired: 7 in]
            n682 = case shown="True" w203 {
              tunnel: w201 -> [_ w205]
              frame False {
              }
              frame True {
                n683 = local write "Message Cluster"(w205) -> ()
              }
            }
          }
          frame #1 {
            n684 = case shown="True" w206 {
              frame False {
              }
              frame True {
                n685 = property on="Digital IO Update" class="Bool (strict)"("Val(Sgnl)"=TRUE ("Value (Signaling)")) -> ()  [unwired: 2 in, 2 out]
              }
            }
            n686 = local write "Setting"(FALSE ("Setting")) -> ()
          }
        }
      }
    }
  }
  n687 = flat-sequence {
    tunnel: w3 -> [_]
    frame #0 {
      n688 = control-ref of="This VI"() -> (w578:refnum<vi>)
      n689 = call "CRYWork Before Step Close.vi"("StepVI Ref"=w578) -> ()  [unwired: 11 in]
    }
    frame #1 {
      n690 = local write "EndFlag"(TRUE ("EndFlag")) -> ()
    }
  }
